vi "Pick&Place_module_cwshih_v0.vi"() -> ()   [LabVIEW 2016]
uses:
  Classes/Controllers/I-O/Copy of NI-DAQ Folder/NI-DAQ.lvclass
  Classes/Controllers/Dispenser/Copy of Ultimus V2 Folder/Ultimus V2.lvclass
  <vilib>/Analysis/coordinate.llb/2D Cartesian Coordinate Rotation (Scalar).vi
  <vilib>/Utility/file.llb/Read Delimited Spreadsheet (DBL).vi
  <vilib>/Utility/file.llb/Write Delimited Spreadsheet (DBL).vi
  Classes/Controllers/Motion/Copy of Motion Folder/Motion.lvclass
  Classes/Controllers/Camera/Copy of Controller Folder/Controller.lvclass
  <vilib>/Analysis/NI_AALPro.lvlib
panel:
  in  "pick up tool measure-start position":dbl[][](array[numeric])=[[147.788, 950.417, 41.7586, -0.0547592], [928.094, 802.097, 34.9367, -0.0626817]]
  out "Array 2":dbl[][](array[numeric])
  out "Measured PickupTool position":dbl[][](array[numeric])
  in  "sampe vacuum":i32[](array[numeric])=[13, 19]
  in  "VacChannel for sample":i32=1
  in  "Values":bool[](array[boolean])=[FALSE, FALSE]
  in  "TrayVaccum":bool
  in  "check height? 2":bool
  in  "check height?":bool
  out "Needle parking position":dbl[](array[numeric])
  out "GlueBox":dbl[][](array[numeric])
  out "appended array":dbl[][](array[numeric])
  in  "chip placement height compensation":dbl=-0.38 format="%#_13g"
  out "Array":dbl[][](array[numeric])
  in  "Sensor A/B":bool
  out "Gantry current position":dbl[](array[numeric])
  in  "READ Position":bool
  in  "Needle Height Compenstation\n(glue gap)":dbl=0.34
  in  "Needle Alignment":bool
  in  "Parking position":dbl[](array[numeric])=[625.0, 625.0, 0.0, 0.01]
  in  "GOTO":bool
  in  "Default Pickup Tool Position":dbl[][](array[numeric])=[[147.788, 950.417, 41.7586, -0.0547592], [928.094, 802.097, 34.9367, -0.0626817]]
  in  "Number of Chips/Sensors \nto be assembled":i32=1
  in  "Default HDI alignment \nmark position":dbl[](array[numeric])=[292.478, 992.407, 78.997, -0.0002369]
  in  "Default HDI size":dbl[](array[numeric])=[24.356, 231.316, -0.0919974, -0.0002369]
  out "# of tasks excuted":i32
  out "Chips on tray position":dbl[][](array[numeric])
  out "measured HDI size":dbl[](array[numeric])
  in  "Chip tray":dbl[](array[numeric])=[388.127, 634.888, 84.693, -0.0231917]
  out "Sample position \non HDI":dbl[][](array[numeric])
  in  "Inititalize":bool
  in  "Pick and place":bool
  in  "Deposit Glue":bool
  in  "Measure Pickup Tools":bool
  in  "Measure Samples on tray":bool
  out "default chip and sensor position w.r.t. 1st mark":dbl[][](array[numeric])
  in  "Assembly Type":bool=TRUE
  in  "Stop":bool
  in  "Measure HDI":bool
  out "Measure HDI top-left":dbl[](array[numeric])
  # "Sensor Tray \nVacuum Channel"
  # "Chips"
  # "Sensor 0.3 -> 200 micron glue thickness\nChips 0.34-> 150 micron glue thickness"
  # "Sensors"
  # "Sensor B short"
  # "Sensors B\n(Short)"
  # "Sensors A\n(Long)"
  # "Sensor A long"
  # "Chips : -0.37-> 60 micron height gap\nSensors (feet stops the lowering)"
  # "ACTIONS"
  # "HDI infomation"
  # "chips use channel 0, 2\nsensors use channel 0, 1"
  # "sensor height 69.8471\nchip height 84.693"
  # "Pick and Place"
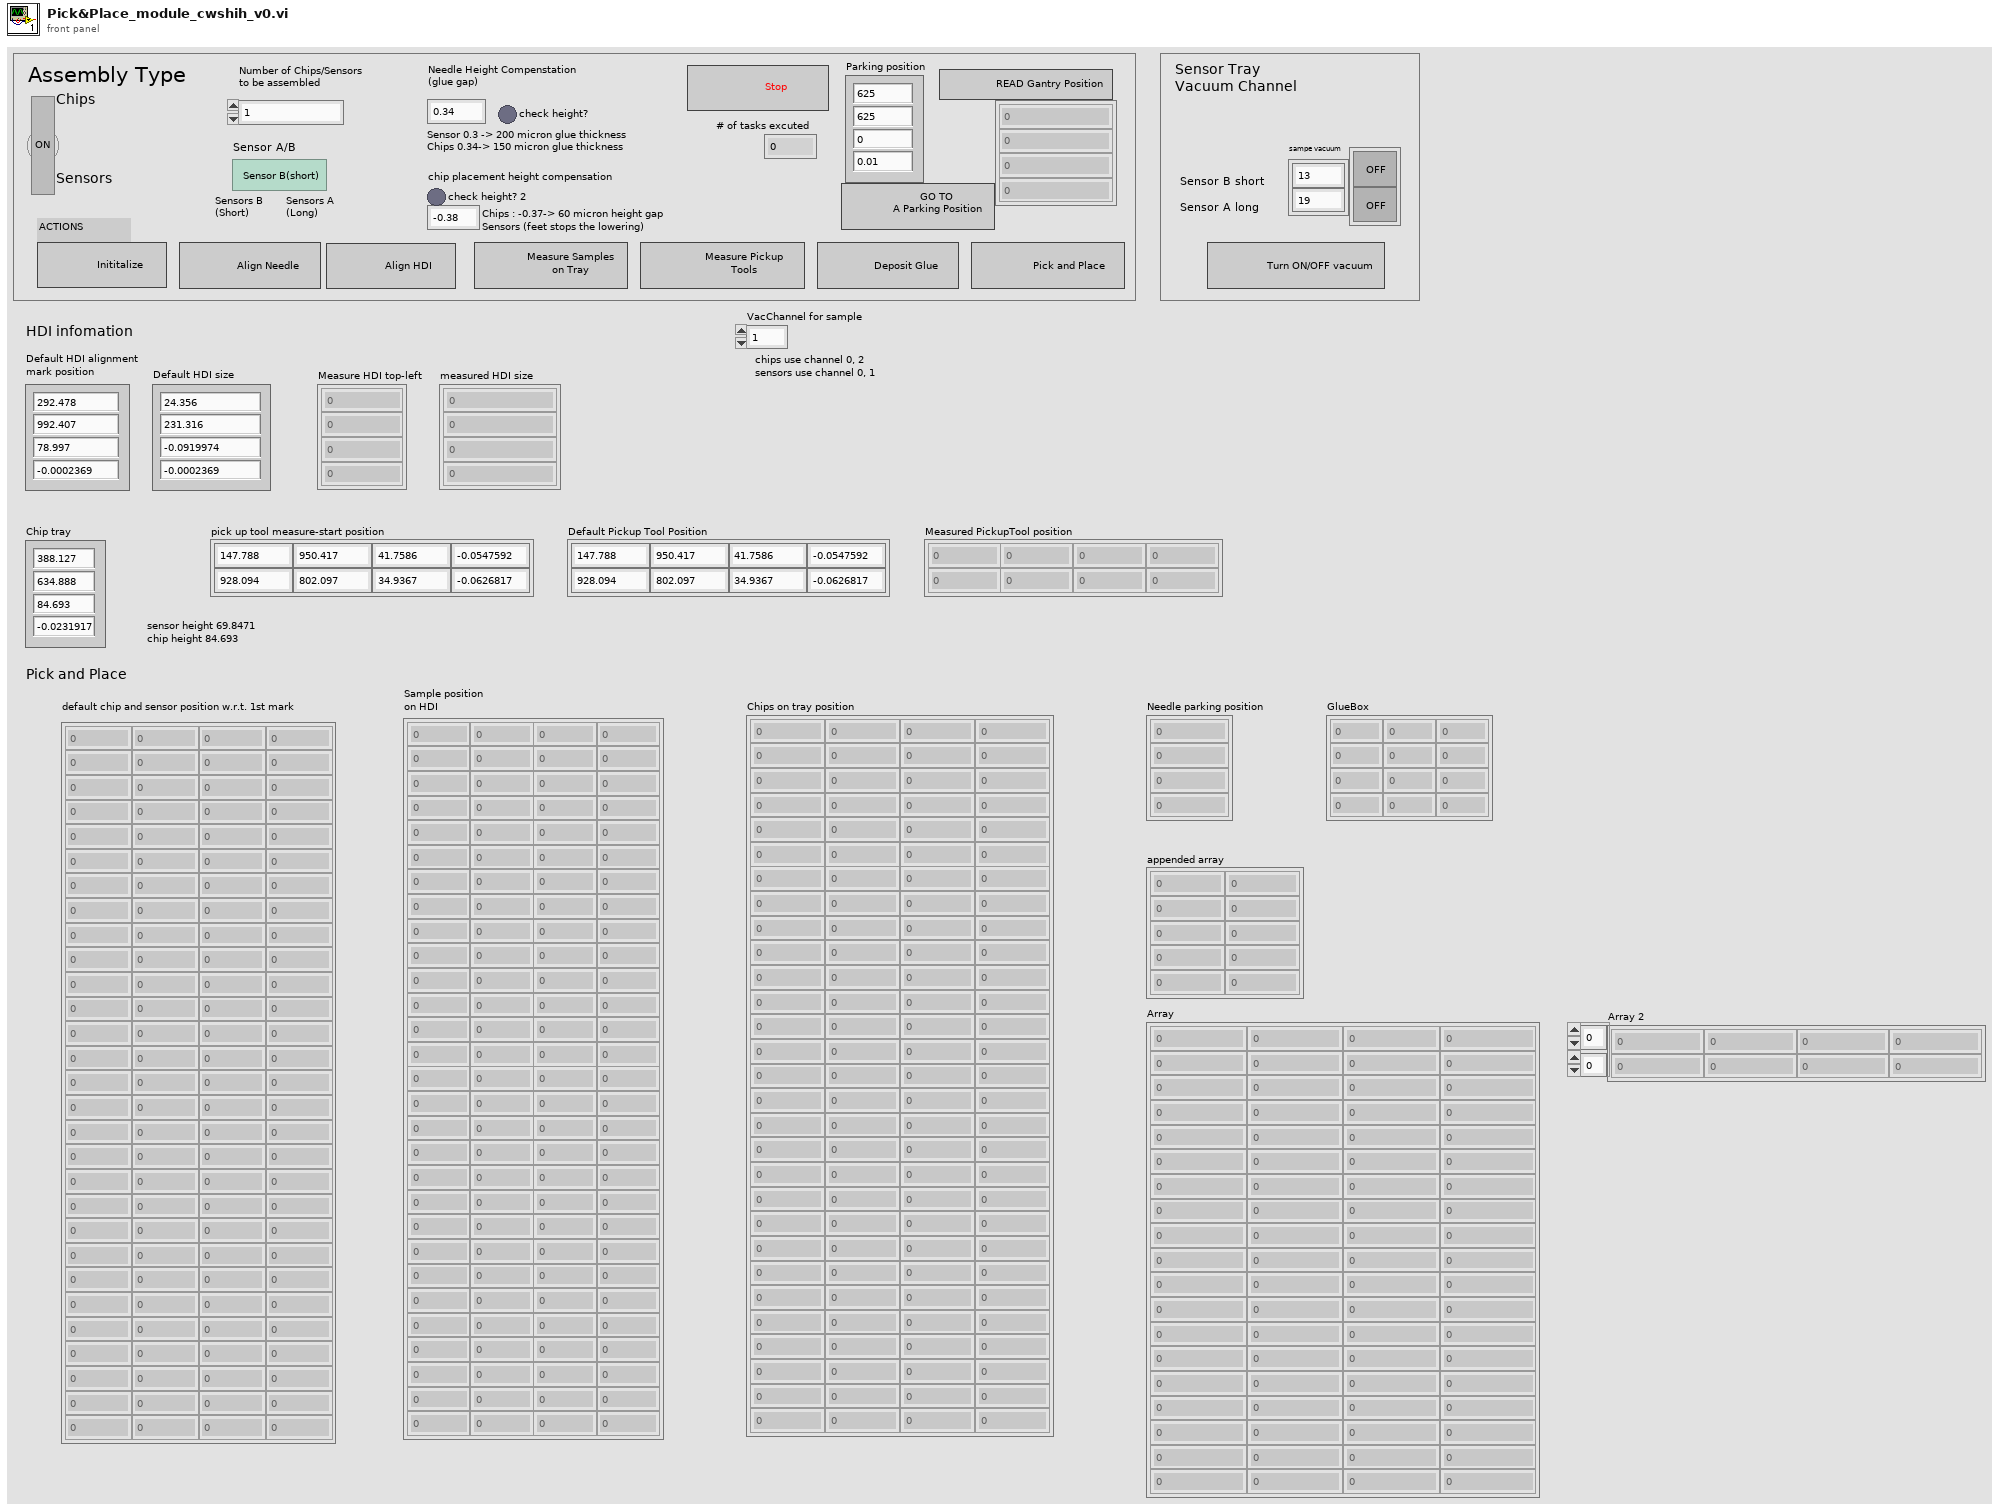
[diagram p1: front panel]
types:
  T1 = typedef "Controller.lvclass/Controllers.ctl" = cluster{"Copy of Motion.lvclass":refnum<class "Motion.lvclass">, "Copy of I-O.lvclass":refnum<class "I-O.lvclass">, "Copy of Dispenser.lvclass":refnum<class "Dispenser.lvclass">}
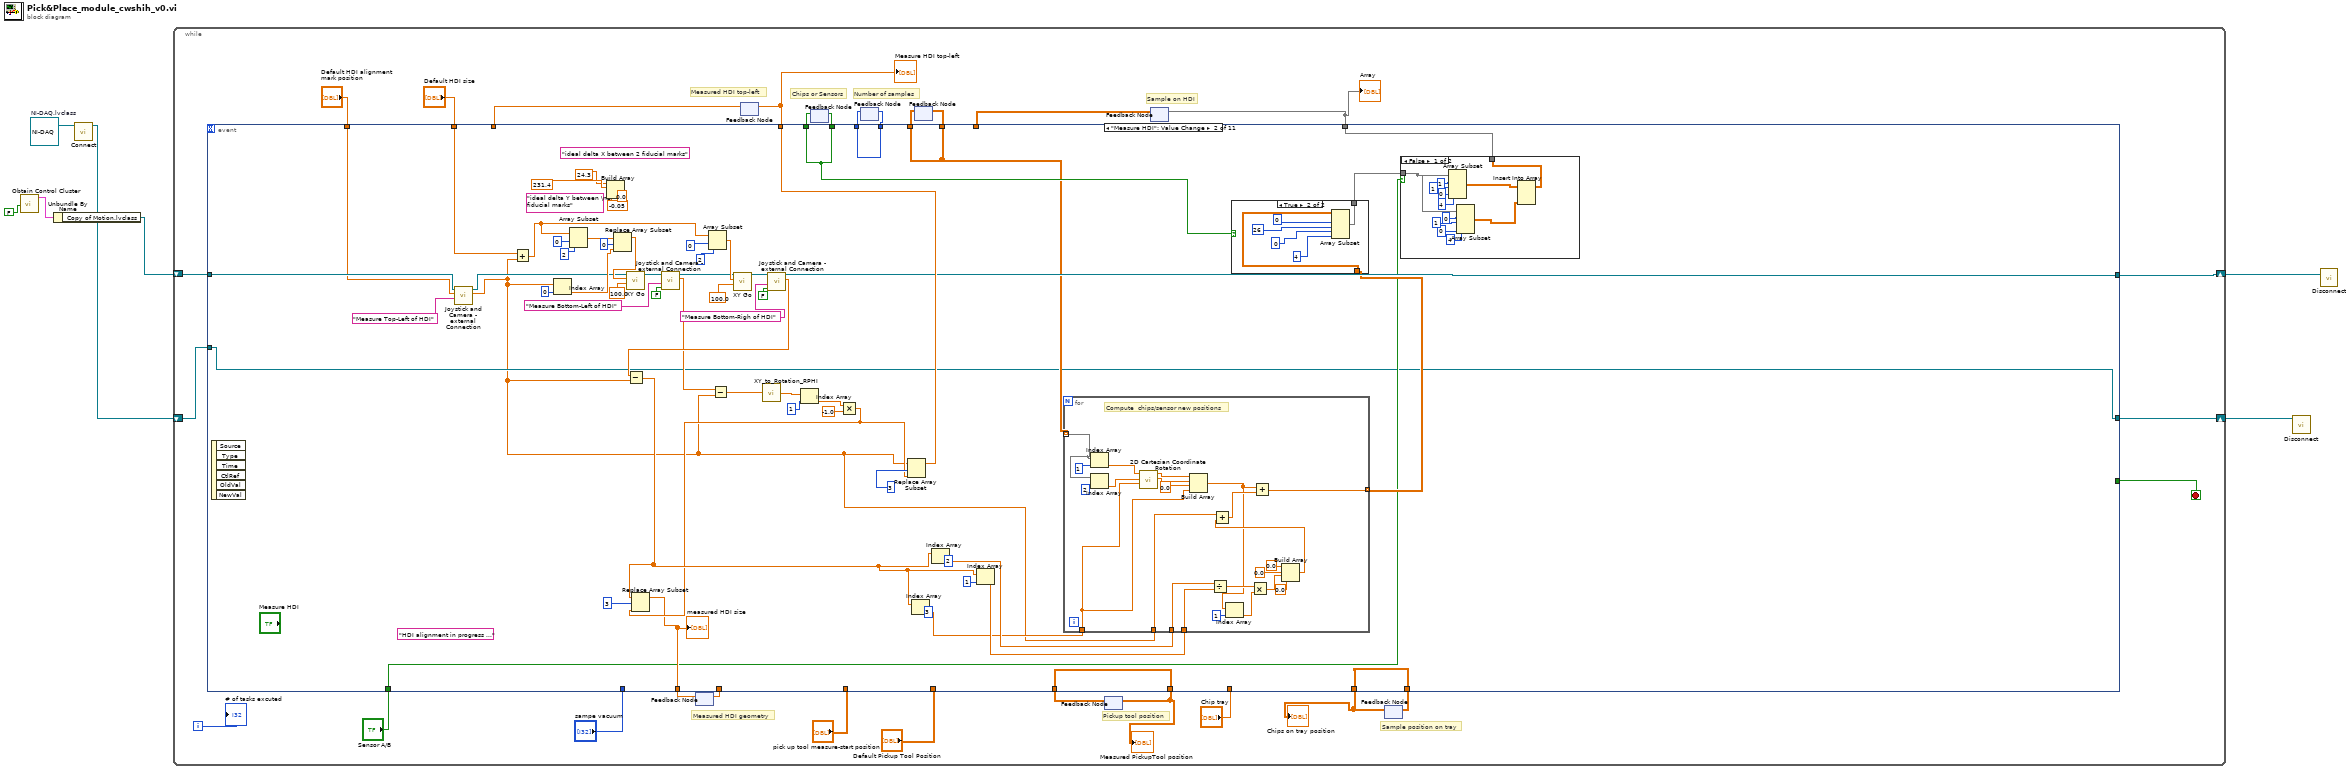
[diagram p0: block diagram]
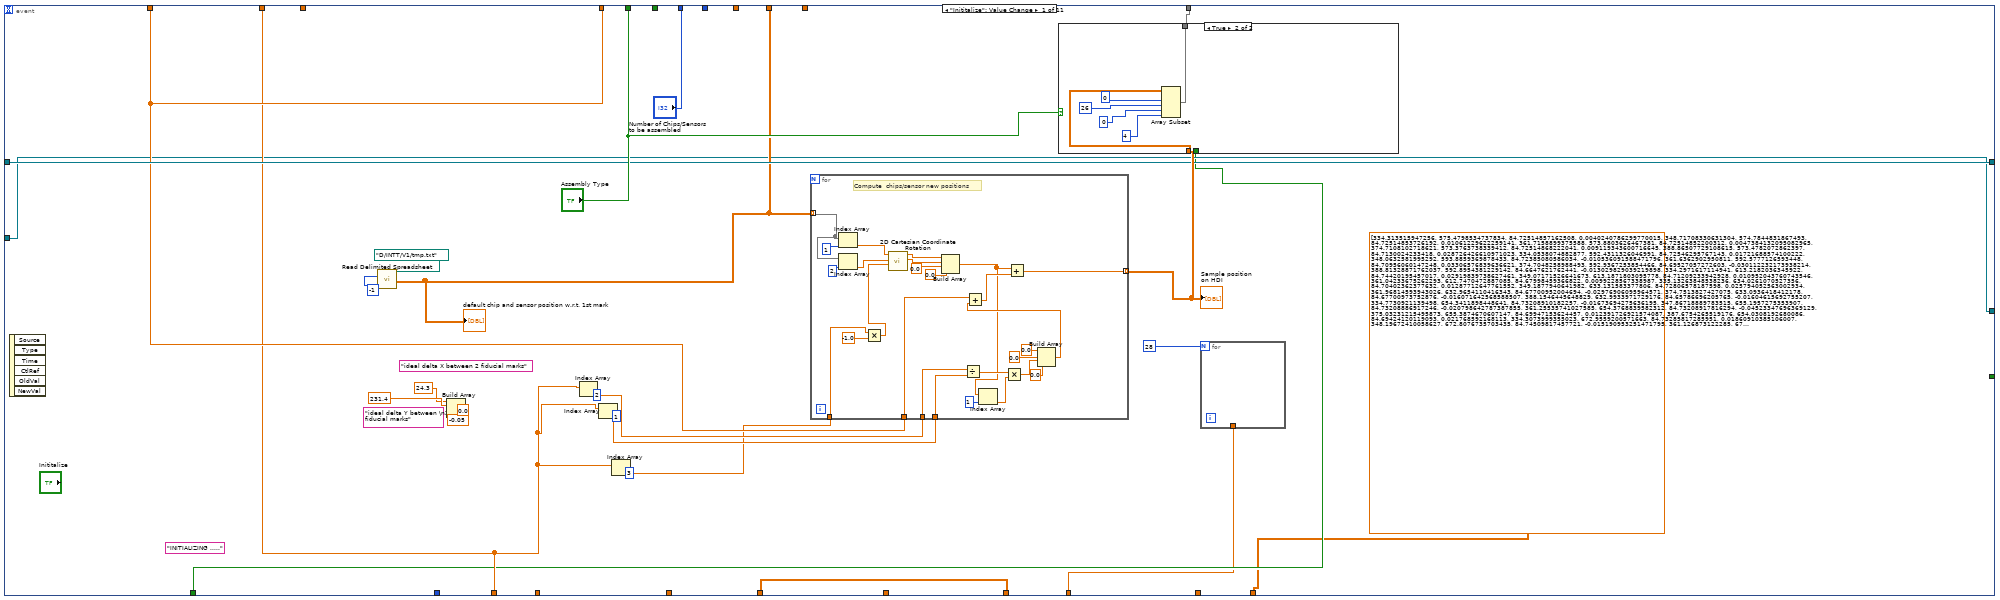
[diagram p2: hidden frame]
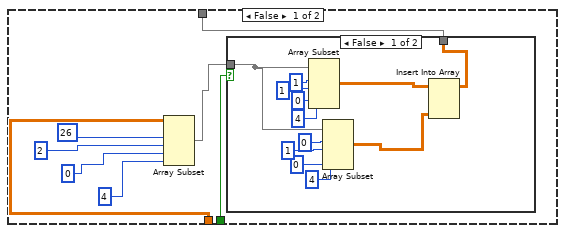
[diagram p3: hidden frame]
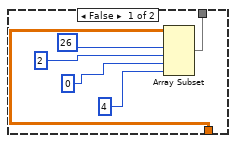
[diagram p6: hidden frame]
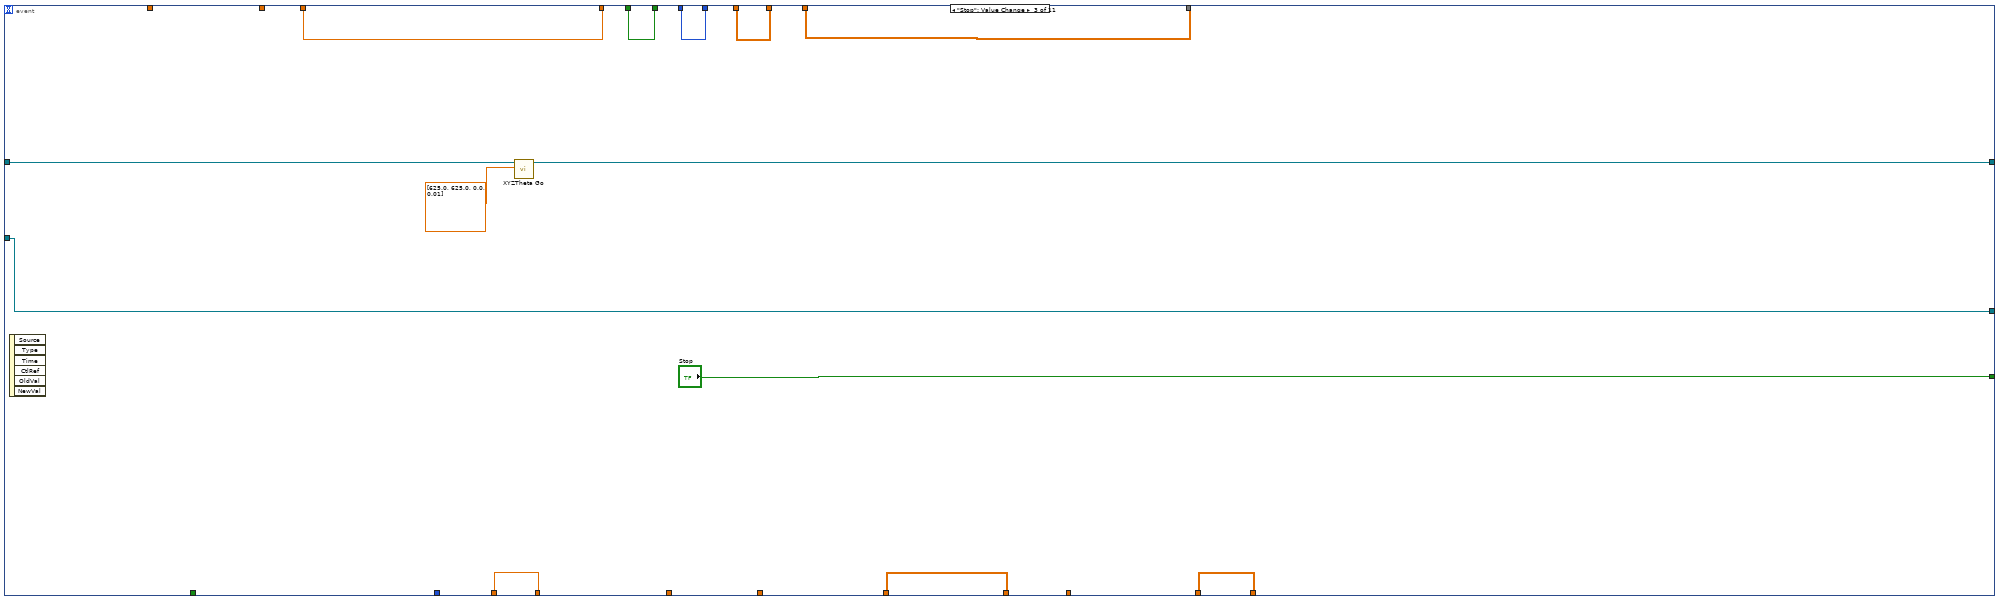
[diagram p7: hidden frame]
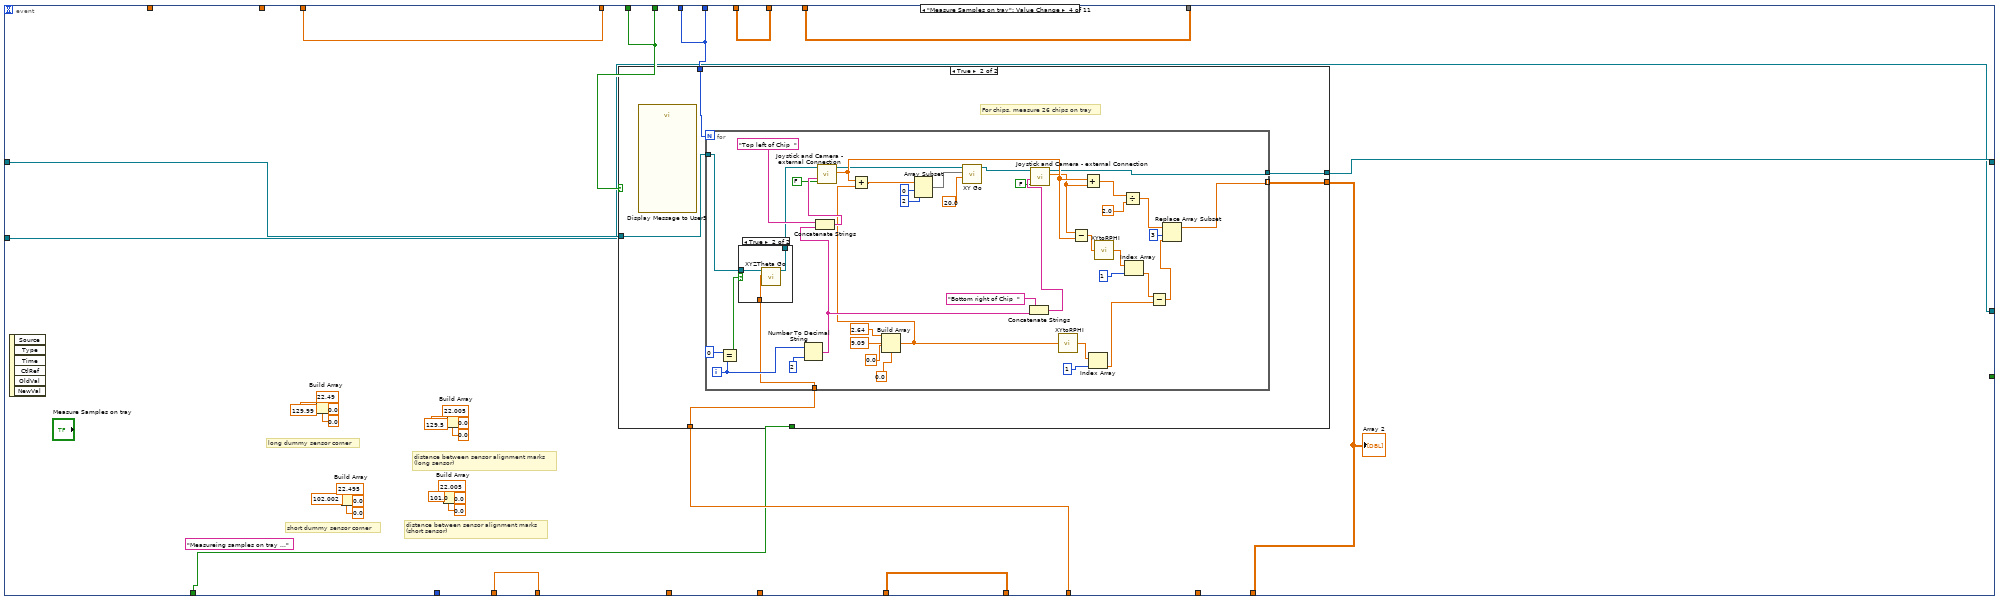
[diagram p8: hidden frame]
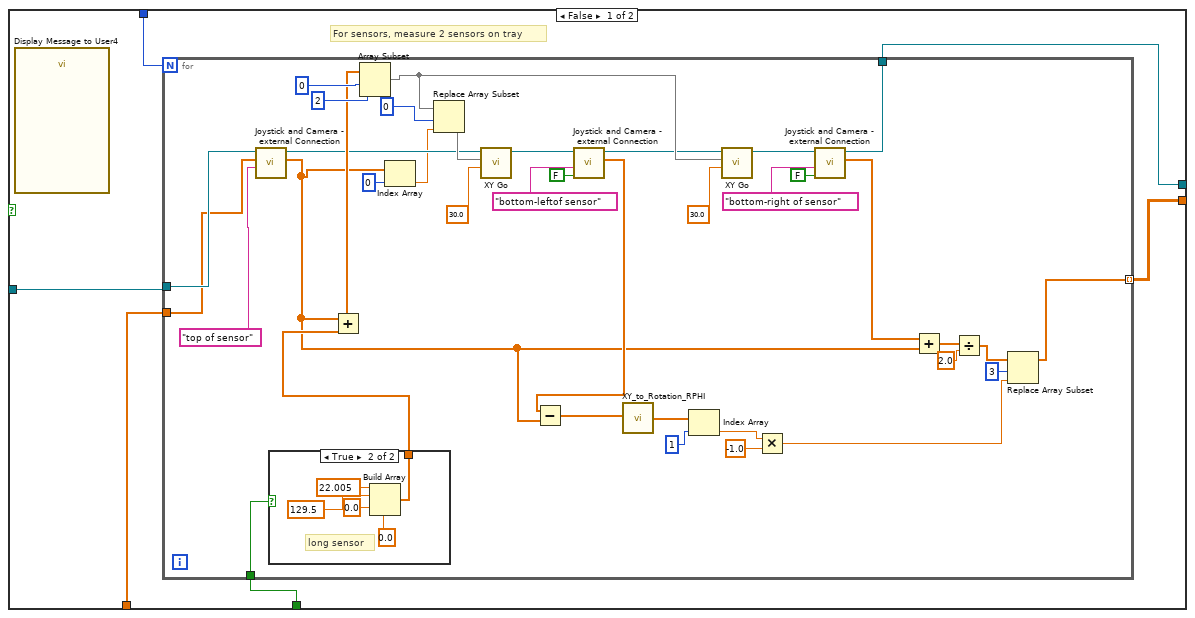
[diagram p9: hidden frame]
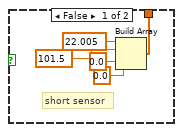
[diagram p10: hidden frame]
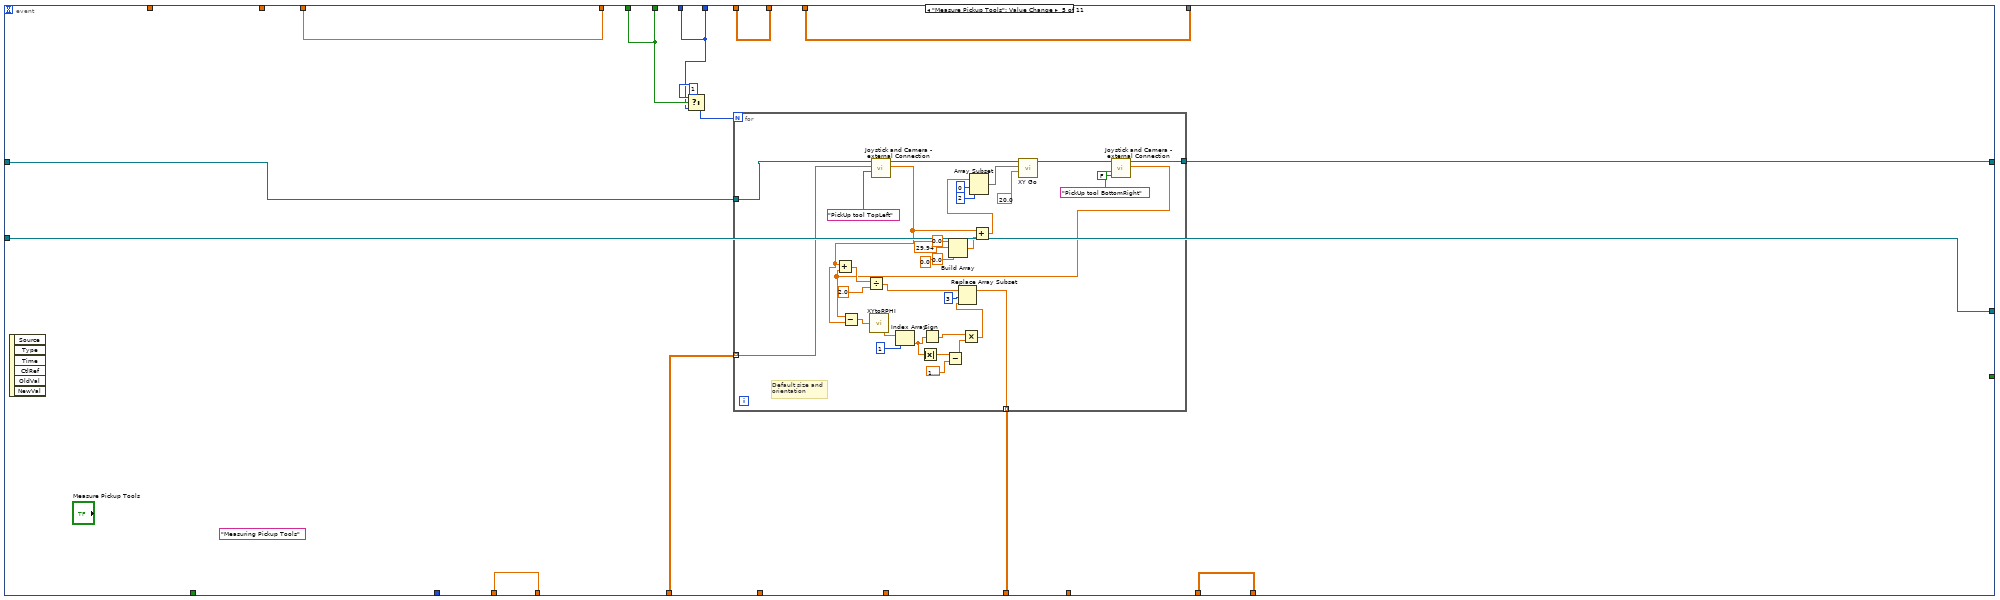
[diagram p12: hidden frame]
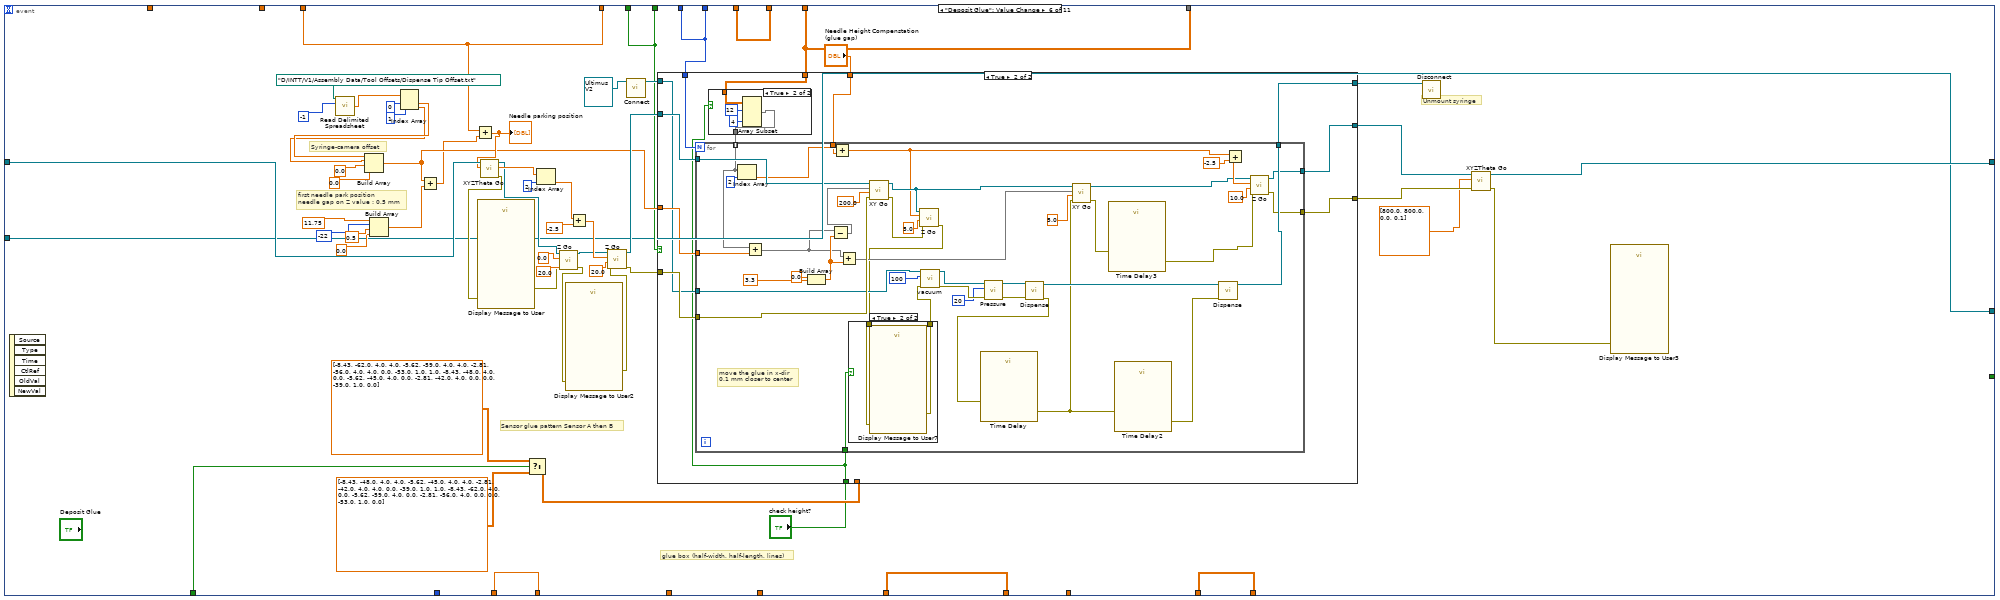
[diagram p13: hidden frame]
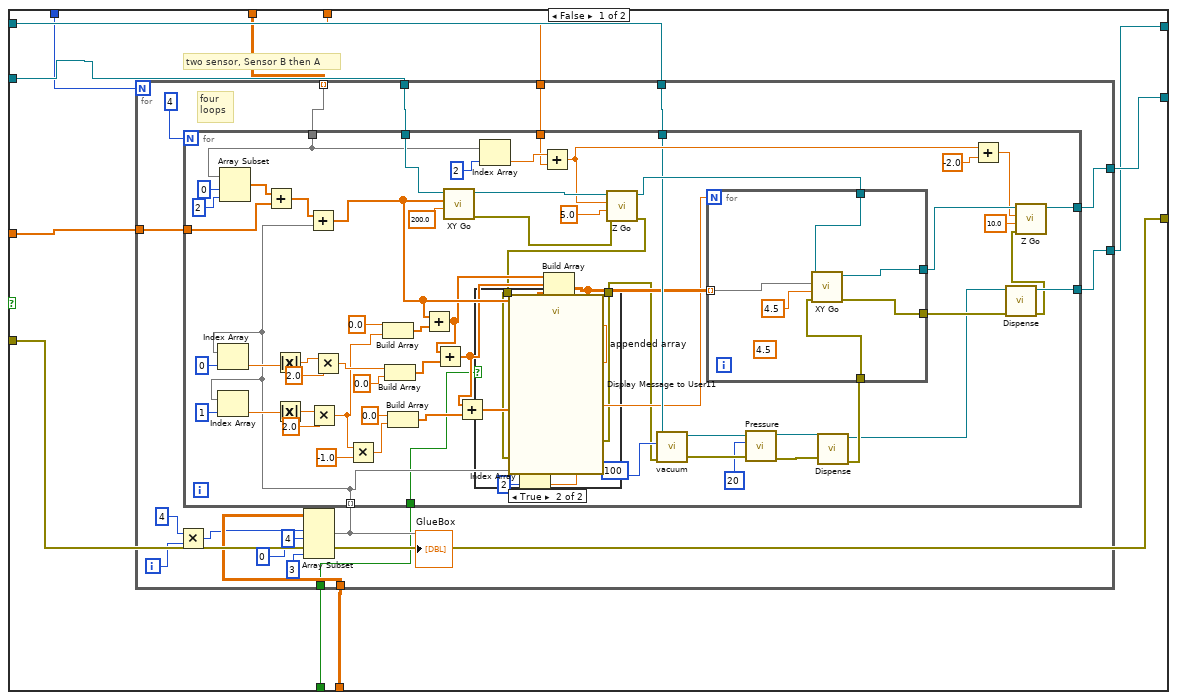
[diagram p14: hidden frame]
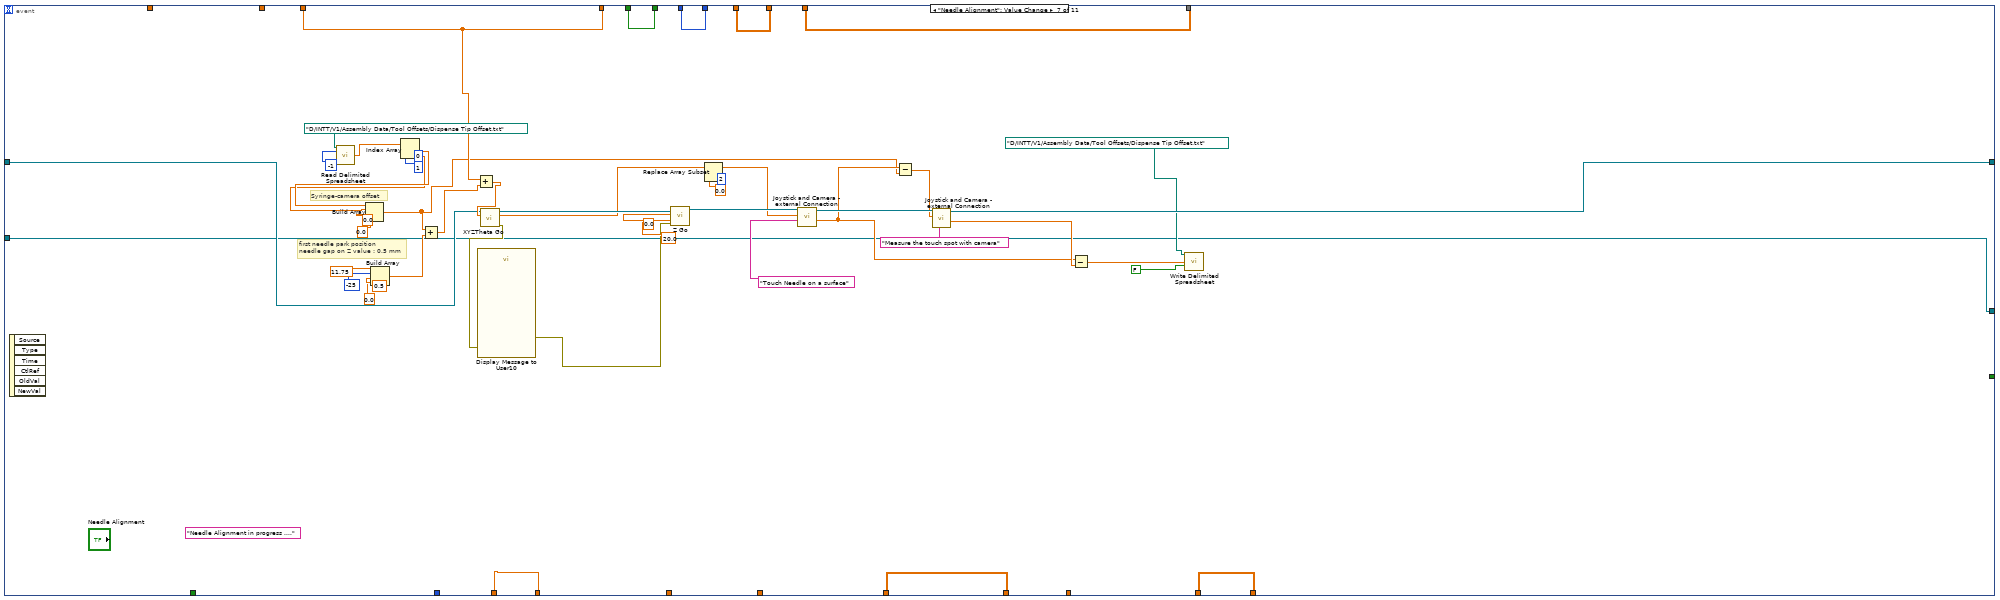
[diagram p18: hidden frame]
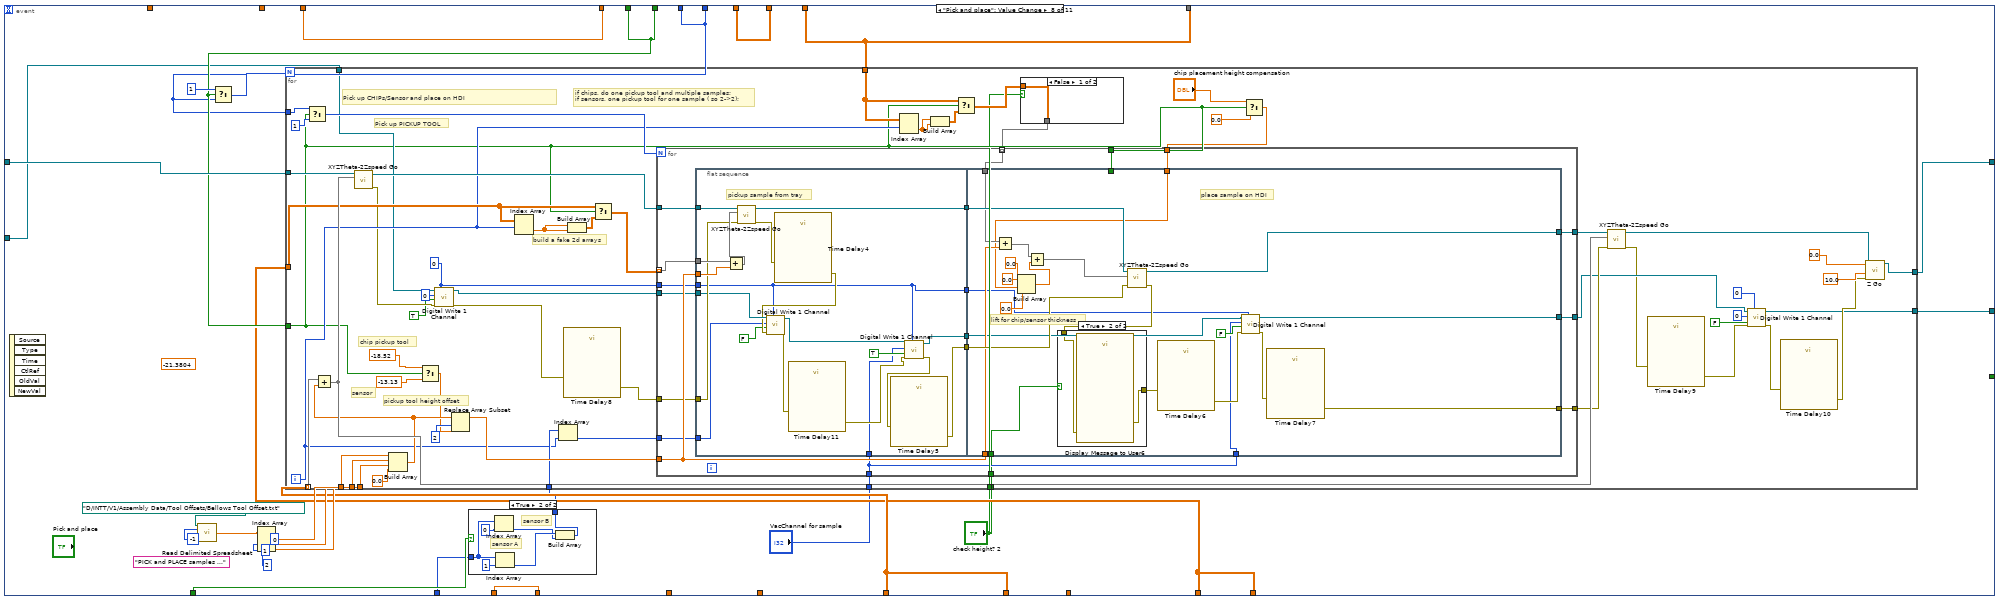
[diagram p19: hidden frame]
diagram:
  w3 = refnum<class "NI-DAQ.lvclass"> refnum  # NI-DAQ.lvclass
  n1 = call "Obtain Control Cluster.vi"("I/O"=FALSE) -> ("Control Out"=w7:T1)  [unwired: 10 in]
  n2 = Unbundle By Name(w7) -> ("Copy of Motion.lvclass"=w5:refnum<class "Motion.lvclass">)
  n3 = call-dynamic "Connect.vi"("NI-DAQ in"=w3) -> ("NI-DAQ out"=w2:refnum<class "NI-DAQ.lvclass">)  [unwired: 9 in, 1 out]
  n4 = while {
    shift-right: [w25] -> w4
    shift-left: w5 -> [w36]
    shift-right: [w12] -> w1
    shift-left: w2 -> [w13]
    i -> [w24]
    stop <- w35 stop-if-true
    # "Pickup tool position"
    # "Chips or Sensors"
    # "Number of samples"
    # "Measured HDI geometry"
    # "Sample position on tray"
    # "Measured HDI top-left"
    # "Sample on HDI"
    n5 = feedback #1() -> (w31:dbl[])  [unwired: 1 in]
    n6 = feedback #2() -> (w33:dbl[])  [unwired: 1 in]
    n7 = feedback #3() -> (w28:bool)  [unwired: 1 in]
    n8 = feedback #4() -> (w23:i32)  [unwired: 1 in]
    n9 = feedback #5() -> (w18:dbl[][])  [unwired: 1 in]
    n10 = feedback #6() -> (w26:dbl[][])  [unwired: 1 in]
    n11 = feedback #7() -> (w30:dbl[][])  [unwired: 1 in]
    n12 = feedback #8() -> (w16:dbl[][])  [unwired: 1 in]
    "Chips on tray position" <- w16
    n13 = event shown="[1] \"Measure HDI\": Value Change" {
      selector: _ -> [_ _ _ _ _ _ _ _ _ _ _]
      dyn-events: _ -> [_ _ _ _ _ _ _ _ _ _ _]
      timeout: _ -> [_ _ _ _ _ _ _ _ _ _ _]
      tunnel: w36 -> [w49 w120 w236 w265 w383 w450 w654 w709 w850 w871 w885]
      tunnel: [_ _ "Stop" _ _ _ _ _ _ _ _] -> w35
      tunnel: [w46 w173 w229 w259 w375 w431 w662 w692 w859 w865 w881] -> w34
      tunnel: w33 -> [_ _ w229 w259 w375 w431 w662 w692 w859 w865 w881]
      tunnel: ["Assembly Type" w166 w233 w263 w379 w434 w661 w698 w858 w866 w882] -> w29
      tunnel: [w44 w125 w228 w258 w374 w427 w657 w691 w854 w864 w880] -> w32
      tunnel: w31 -> [_ _ w228 w258 w374 w427 w657 w691 w854 w864 w880]
      tunnel: [w41 w123 w230 w260 w377 w433 w658 w697 w855 w869 w884] -> w14
      tunnel: w30 -> [_ _ w230 w260 w377 w433 w658 w697 w855 w869 w884]
      tunnel: w28 -> [_ w166 w233 w263 w379 w434 w661 w698 w858 w866 w882]
      tunnel: w23 -> [_ w163 w232 w262 w378 w432 w660 w694 w857 w867 w877]
      tunnel: [dbl[][] [[334.313515947256, 575.4798534737834, 84.72514857162508, 0.0040240786299770015], [348.71708330631304, 574.7844831867493, 84.72514853726192, 0.01061229622259141], [361.7158899375588, 573.8803626467381, 84.72514852200312, 0.0047384132095082965], [374.7108102718621, 573.3763738339412, 84.72514868222041, 0.009119343600716645], [388.86507729108615, 573.4782072862397, 84.7130024233418, 0.028726426610971023], [334.0538074882877, 592.4311326046991, 84.72546295767143, 0.01721688574100222], [348.0632581995292, 593.8859369878433, 84.72385080586034, -0.010536091588471796], [361.6362902950811, 592.5777126593448, 84.70956060147248, 0.03306576839636621], [374.7048258988493, 592.9367253854466, 84.69527057272603, -0.030112232173938214], [388.81328871762037, 592.8954381229142, 84.6647621762441, -0.013029829039219898], [334.2971617114941, 613.2182036345922, 84.74420195457017, 0.02919839738627461], [349.07171526641673, 613.1871803095778, 84.71209233942928, 0.010952043760743546], [361.04233675262293, 612.7470472887085, 84.67998459366822, 0.0099228567338987], [335.13263848538236, 634.0261070527356, 84.70402362377632, 0.01287712647761552], [349.1877940641982, 633.131583377806, 84.72806578187598, 0.025794052563002934], [361.96814593943026, 632.9654110416343, 84.67700952004694, -0.02976906095964571], [374.7513827427075, 633.0936418412178, 84.67700973752876, -0.016071642568588507], [388.1546445648829, 632.9933971729176, 84.65786696205765, -0.01604615692755207], [334.7730921139498, 654.3411898448641, 84.73208910182257, -0.01673694275636195], [347.86718889783515, 655.1957275353907, 84.73208886917246, -0.020798642787387855], [361.25535741027585, 654.3768839582312, 84.73208917816294, -0.04523347696369129], [375.03231215495873, 655.3874670607147, 84.69947153624457, 0.012391726921574087], [387.6754265519176, 654.0308192680086, 84.69424120119093, 0.021768592168113], [334.3073999355023, 672.9559200571663, 84.73285817285951, 0.01860910385106007], [348.19672410058627, 672.8076735703435, 84.74509817457721, -0.015190953251471795], [361.126873122285, 672.7320047678002, 84.74509773207234, -0.005257017136958586]] ("Chips on tray position") w161 w226 w238 w373 w429 w655 w695 w852 w862 w878] -> w27
      tunnel: w16 -> [_ w161 w226 _ w373 w429 w655 w695 w852 w862 w878]
      tunnel: [w39 w162 w227 w257 w382 w428 w656 w696 w853 w863 w879] -> w8
      tunnel: w26 -> [_ w162 w227 w257 _ w428 w656 w696 w853 w863 w879]
      tunnel: [w49 w172 w234 w264 w381 w435 w646 w699 w849 w870 w885] -> w25
      tunnel: ["Number of Chips/Sensors \nto be assembled" w163 w232 w262 w378 w432 w660 w694 w857 w867 w877] -> w22
      tunnel: "Default HDI alignment \nmark position" -> [w46 w116 _ _ _ _ _ _ _ _ _]
      tunnel: "Default HDI size" -> [w44 w171 _ _ _ _ _ _ _ _ _]
      tunnel: [w47 w164 w231 w261 w376 w426 w659 w693 w856 w868 w883] -> w19
      tunnel: w18 -> [_ w164 w231 w261 w376 w426 w659 w693 w856 w868 w883]
      tunnel: "Chip tray" -> [w38 _ _ w256 _ _ _ _ _ _ _]
      tunnel: "Sensor A/B" -> [w40 w122 _ w247 _ w425 _ w690 _ _ _]
      tunnel: w13 -> [w42 w121 w224 w237 w372 w419 w637 w687 w851 w860 w876]
      tunnel: [w42 w121 w224 w237 w372 w419 w637 w688 w851 w860 w875] -> w12
      tunnel: "sampe vacuum" -> [_ _ _ _ _ _ _ w685 _ _ w872]
      tunnel: "Default Pickup Tool Position" -> [w39 _ _ _ _ _ _ _ _ _ _]
      tunnel: "pick up tool measure-start position" -> [_ _ _ _ w371 _ _ _ _ _ _]
      event "Inititalize": Value Change {
        (unwired) "INITIALIZING ....." ("String")
        (unwired) "ideal delta Y between \n2 fiducial marks"
        (unwired) "ideal delta X between 2 fiducial marks"
        n14 = event-data() -> ()  [unwired: 1 in, 6 out]
        n15 = call-poly <vilib>:"Read Delimited Spreadsheet.vi"("file path (dialog if empty)"=path "D:/INTT/V1/tmp.txt", "number of rows (all:-1)"=-1) -> ("all rows"=w47:dbl[][])  [unwired: 8 in, 5 out]
        "default chip and sensor position w.r.t. 1st mark" <- w47
        n16 = Build Array(24.3 ("y"), 231.4 ("y"), 0.0 ("element"), -0.05 ("element")) -> ()  [unwired: 1 out]
        n17 = Index Array(array=w44, index=2) -> (element=w58:dbl)
        n18 = Index Array(array=w44, index=1) -> (element=w57:dbl)
        n19 = Index Array(array=w44, index=3) -> (element=w43:dbl)
        n20 = for {
          tunnel: w47 -> [w108] mode=indexing
          tunnel: w43 -> [w91]
          tunnel: w46 -> [w100]
          tunnel: [w107] -> w51 mode=indexing
          tunnel: w58 -> [w106]
          tunnel: w57 -> [w97]
          # "Compute  chips/sensor new positions"
          n21 = Index Array(array=w108, index=1) -> (element=w112:dbl)
          n22 = Index Array(array=w108, index=2) -> (element=w111:dbl)
          n23 = Multiply(x=w91, y=-1.0) -> (x*y=w90:dbl)
          n24 = call-poly <vilib>:"2D Cartesian Coordinate Rotation.vi"("theta"=w90, "y"=w111, "x"=w112) -> ("y out"=w114:dbl, "x out"=w113:dbl)  [unwired: 6 in, 1 out]
          n25 = Build Array(w113, w114, 0.0 ("element"), 0.0 ("element")) -> (w94:dbl[])
          n26 = Divide(x=w106, y=w97) -> (x/y=w105:dbl)
          n27 = Index Array(array=w94, index=1) -> (element=w95:dbl)
          n28 = Multiply(x=w105, y=w95) -> (x*y=w101:dbl)
          n29 = Build Array(0.0 ("element"), 0.0 ("element"), w101, 0.0 ("element")) -> (w99:dbl[])
          n30 = Add(x=w100, y=w99) -> (x+y=w98:dbl[])
          n31 = Add(x=w94, y=w98) -> (x+y=w107:dbl[])
        }
        "Sample position \non HDI" <- w51
        n32 = case shown="True" "Assembly Type" {
          tunnel: w51 -> [w66 w86]
          tunnel: [w64 w84] -> w41
          tunnel: w40 -> [w63 _]
          frame False {
            n33 = Array Subset(array=w66, index (row)=26 ("index"), length (row)=2 ("length"), index (col)=0, length (col)=4 ("length")) -> (w65:dbl[][])
            n34 = case shown="False" w63 {
              tunnel: w65 -> [w74 w83]
              tunnel: [w71 w83] -> w64
              frame False {
                n35 = Array Subset(array=w74, index (row)=1 ("index"), length (row)=1 ("length"), index (col)=0 ("index"), length (col)=4 ("length")) -> (w73:dbl[][])
                n36 = Array Subset(array=w74, index (row)=0 ("index"), length (row)=1 ("length"), index (col)=0 ("index"), length (col)=4 ("length")) -> (w72:dbl[][])
                n37 = Insert Into Array(array=w73, new element=w72) -> (w71:dbl[][])  [unwired: 2 in]
              }
              frame True {
              }
            }
          }
          frame True {
            n38 = Array Subset(array=w86, index (row)=0 ("index"), length (row)=26 ("length"), index (col)=0, length (col)=4 ("length")) -> (w84:dbl[][])
          }
        }
        n39 = for {
          N: 28 -> [_]
          tunnel: w38 -> [_]
        }
      }
      event "Measure HDI": Value Change {
        (unwired) "ideal delta Y between \n2 fiducial marks"
        (unwired) "ideal delta X between 2 fiducial marks"
        (unwired) "HDI alignment in progress ..." ("String")
        n40 = event-data() -> ()  [unwired: 1 in, 6 out]
        n41 = call "Joystick and Camera - external Connection.vi"("Motion in"=w120, "XYZTheta"=w116, "Measurement Point"="Measure Top-Left of HDI") -> ("Motion out"=w119:refnum<class "Motion.lvclass">, "Sum"=w118:dbl[])  [unwired: 4 in, 2 out]
        n42 = Add(x=w171, y=w118) -> (x+y=w143:dbl[])
        n43 = Index Array(array=w118, index=0) -> (element=w132:dbl)
        n44 = Array Subset(array=w143, index=0, length=2) -> (w142:dbl[])
        n45 = Build Array(24.3 ("y"), 231.4 ("y"), 0.0 ("element"), -0.05 ("element")) -> ()  [unwired: 1 out]
        n46 = Replace Array Subset(array=w142, new element=w132, index=0) -> (w140:dbl[])
        n47 = call-dynamic "XY Go.vi"("Speed"=100.0, "XY"=w140, "Motion in"=w119) -> ("Motion out"=w147:refnum<class "Motion.lvclass">)  [unwired: 7 in, 1 out]
        n48 = call "Joystick and Camera - external Connection.vi"("Motion in"=w147, "Measurement Point"="Measure Bottom-Left of HDI", "Inital GO"=FALSE) -> ("Motion out"=w139:refnum<class "Motion.lvclass">, "Sum"=w131:dbl[])  [unwired: 4 in, 2 out]
        n49 = Array Subset(array=w143, index=0, length=2) -> (w153:dbl[])
        n50 = Subtract(x=w131, y=w118) -> (x-y=w138:dbl[])
        n51 = call-dynamic "XY Go.vi"("Speed"=100.0, "XY"=w153, "Motion in"=w139) -> ("Motion out"=w157:refnum<class "Motion.lvclass">)  [unwired: 7 in, 1 out]
        n52 = call "XY_to_Rotation_RPHI.vi"("X-Y"=w138) -> ("r-phi"=w135:dbl[])
        n53 = call "Joystick and Camera - external Connection.vi"("Motion in"=w157, "Measurement Point"="Measure Bottom-Righ of HDI", "Inital GO"=FALSE) -> ("Motion out"=w172:refnum<class "Motion.lvclass">, "Sum"=w175:dbl[])  [unwired: 4 in, 2 out]
        n54 = Subtract(x=w175, y=w118) -> (x-y=w128:dbl[])
        n55 = Index Array(array=w135, index=1) -> (element=w129:dbl)
        n56 = Multiply(x=w129, y=-1.0) -> (x*y=w126:dbl)
        n57 = Replace Array Subset(array=w128, new element=w126, index=3) -> (w125:dbl[])
        "measured HDI size" <- w125
        n58 = Replace Array Subset(array=w118, new element=w126, index=3) -> (w173:dbl[])
        n59 = Index Array(array=w128, index=3) -> (element=w159:dbl)
        n60 = Index Array(array=w128, index=2) -> (element=w168:dbl)
        n61 = Index Array(array=w128, index=1) -> (element=w167:dbl)
        n62 = for {
          tunnel: w164 -> [w216] mode=indexing
          tunnel: w159 -> [w201]
          tunnel: w118 -> [w208]
          tunnel: [w215] -> w165 mode=indexing
          tunnel: w168 -> [w214]
          tunnel: w167 -> [w205]
          # "Compute  chips/sensor new positions"
          n63 = Index Array(array=w216, index=1) -> (element=w220:dbl)
          n64 = Index Array(array=w216, index=2) -> (element=w219:dbl)
          n65 = call-poly <vilib>:"2D Cartesian Coordinate Rotation.vi"("theta"=w201, "y"=w219, "x"=w220) -> ("y out"=w222:dbl, "x out"=w221:dbl)  [unwired: 6 in, 1 out]
          n66 = Build Array(w221, w222, 0.0 ("element"), w201) -> (w202:dbl[])
          n67 = Divide(x=w214, y=w205) -> (x/y=w213:dbl)
          n68 = Index Array(array=w202, index=1) -> (element=w203:dbl)
          n69 = Multiply(x=w213, y=w203) -> (x*y=w209:dbl)
          n70 = Build Array(0.0 ("element"), 0.0 ("element"), w209, 0.0 ("element")) -> (w207:dbl[])
          n71 = Add(x=w208, y=w207) -> (x+y=w206:dbl[])
          n72 = Add(x=w202, y=w206) -> (x+y=w215:dbl[])
        }
        n73 = case shown="True" w166 {
          tunnel: w165 -> [w190 w197]
          tunnel: [w189 w195] -> w124
          frame False {
            n74 = Array Subset(array=w190, index (row)=26 ("index"), length (row)=2 ("length"), index (col)=0, length (col)=4 ("length")) -> (w189:dbl[][])
          }
          frame True {
            n75 = Array Subset(array=w197, index (row)=0 ("index"), length (row)=26 ("length"), index (col)=0, length (col)=4 ("length")) -> (w195:dbl[][])
          }
        }
        n76 = case shown="False" w122 {
          tunnel: w124 -> [w179 w188]
          tunnel: [w176 w188] -> w123
          frame False {
            n77 = Array Subset(array=w179, index (row)=1 ("index"), length (row)=1 ("length"), index (col)=0 ("index"), length (col)=4 ("length")) -> (w178:dbl[][])
            n78 = Array Subset(array=w179, index (row)=0 ("index"), length (row)=1 ("length"), index (col)=0 ("index"), length (col)=4 ("length")) -> (w177:dbl[][])
            n79 = Insert Into Array(array=w178, new element=w177) -> (w176:dbl[][])  [unwired: 2 in]
          }
          frame True {
          }
        }
      }
      event "Stop": Value Change {
        n80 = event-data() -> ()  [unwired: 1 in, 6 out]
        n81 = call "XYZTheta Go.vi"("XYZTheta In"=dbl[] [625.0, 625.0, 0.0, 0.01], "Motion in"=w236) -> ("Motion out"=w234:refnum<class "Motion.lvclass">)  [unwired: 7 in, 2 out]
      }
      event "Measure Samples on tray": Value Change {
        (unwired) "Measureing samples on tray ..." ("String")
        # "long dummy sensor corner"
        # "short dummy sensor corner"
        # "distance between sensor alignment marks\n(short sensor)"
        # "distance between sensor alignment marks\n(long sensor)"
        n82 = event-data() -> ()  [unwired: 1 in, 6 out]
        n83 = Build Array(22.49 ("element"), 129.99 ("element"), 0.0 ("element"), 0.0 ("element")) -> ()  [unwired: 1 out]
        n84 = Build Array(22.495 ("element"), 102.002 ("element"), 0.0 ("element"), 0.0 ("element")) -> ()  [unwired: 1 out]
        n85 = Build Array(22.005 ("element"), 101.0 ("element"), 0.0 ("element"), 0.0 ("element")) -> ()  [unwired: 1 out]
        n86 = Build Array(22.005 ("element"), 129.5 ("element"), 0.0 ("element"), 0.0 ("element")) -> ()  [unwired: 1 out]
        n87 = case shown="True" w263 {
          tunnel: [w267 w324] -> w238
          tunnel: w265 -> [w271 w323]
          tunnel: [w266 w322] -> w264
          tunnel: w262 -> [w270 w321]
          tunnel: w256 -> [w269 w320]
          tunnel: w247 -> [w268 _]
          frame False {
            # "For sensors, measure 2 sensors on tray"
            n88 = call "Display Message to User4"() -> ()  [unwired: 10 in, 2 out]
            n89 = for {
              N: w270 -> [_]
              tunnel: w271 -> [w309]
              tunnel: [w306] -> w266
              tunnel: [w299] -> w267 mode=indexing
              tunnel: w269 -> [w298]
              tunnel: w268 -> [w297]
              n90 = call "Joystick and Camera - external Connection.vi"("Motion in"=w309, "XYZTheta"=w298, "Measurement Point"="top of sensor") -> ("Motion out"=w276:refnum<class "Motion.lvclass">, "Sum"=w273:dbl[])  [unwired: 4 in, 2 out]
              n91 = case shown="True" w297 {
                tunnel: [w310 w316] -> w300
                frame False {
                  # "short sensor"
                  n92 = Build Array(22.005 ("element"), 101.5 ("element"), 0.0 ("element"), 0.0 ("element")) -> (w310:dbl[])
                }
                frame True {
                  # "long sensor"
                  n93 = Build Array(22.005 ("element"), 129.5 ("element"), 0.0 ("element"), 0.0 ("element")) -> (w316:dbl[])
                }
              }
              n94 = Add(x=w273, y=w300) -> (x+y=w286:dbl[])
              n95 = Array Subset(array=w286, index=0, length=2) -> (w287:dbl[])
              n96 = Index Array(array=w273, index=0) -> (element=w272:dbl)
              n97 = Replace Array Subset(array=w287, new element=w272, index=0) -> (w284:dbl[])
              n98 = call-dynamic "XY Go.vi"("Speed"=30.0, "XY"=w284, "Motion in"=w276) -> ("Motion out"=w289:refnum<class "Motion.lvclass">)  [unwired: 7 in, 1 out]
              n99 = call "Joystick and Camera - external Connection.vi"("Motion in"=w289, "Measurement Point"="bottom-leftof sensor", "Inital GO"=FALSE) -> ("Motion out"=w275:refnum<class "Motion.lvclass">, "Sum"=w278:dbl[])  [unwired: 4 in, 2 out]
              n100 = Subtract(x=w278, y=w273) -> (x-y=w283:dbl[])
              n101 = call "XY_to_Rotation_RPHI.vi"("X-Y"=w283) -> ("r-phi"=w282:dbl[])
              n102 = Index Array(array=w282, index=1) -> (element=w279:dbl)
              n103 = call-dynamic "XY Go.vi"("Speed"=30.0, "XY"=w287, "Motion in"=w275) -> ("Motion out"=w295:refnum<class "Motion.lvclass">)  [unwired: 7 in, 1 out]
              n104 = Multiply(x=w279, y=-1.0) -> (x*y=w277:dbl)
              n105 = call "Joystick and Camera - external Connection.vi"("Motion in"=w295, "Measurement Point"="bottom-right of sensor", "Inital GO"=FALSE) -> ("Motion out"=w306:refnum<class "Motion.lvclass">, "Sum"=w303:dbl[])  [unwired: 4 in, 2 out]
              n106 = Add(x=w303, y=w273) -> (x+y=w304:dbl[])
              n107 = Divide(x=w304, y=2.0) -> (x/y=w302:dbl[])
              n108 = Replace Array Subset(array=w302, new element=w277, index=3) -> (w299:dbl[])
            }
          }
          frame True {
            # "For chips, measure 26 chips on tray"
            n109 = call "Display Message to User5"() -> ()  [unwired: 10 in, 2 out]
            n110 = for {
              N: w321 -> [_]
              tunnel: [w353] -> w324 mode=indexing
              tunnel: w323 -> [w337]
              tunnel: [w333] -> w322
              tunnel: w320 -> [w338]
              i -> [w341]
              n111 = Equal?(x=0, y=w341) -> (x = y?=w339:bool)
              n112 = case shown="True" w339 {
                tunnel: w338 -> [_ w370]
                tunnel: w337 -> [w367 w369]
                tunnel: [w367 w368] -> w336
                frame False {
                }
                frame True {
                  n113 = call "XYZTheta Go.vi"("XYZTheta In"=w370, "Motion in"=w369) -> ("Motion out"=w368:refnum<class "Motion.lvclass">)  [unwired: 7 in, 2 out]
                }
              }
              n114 = Number To Decimal String(number=w341, width (-)=i16 2) -> (decimal integer string=w357:string)
              n115 = Concatenate Strings("Top left of Chip  " ("string"), w357) -> (w351:string)
              n116 = call "Joystick and Camera - external Connection.vi"("Motion in"=w336, "Measurement Point"=w351, "Inital GO"=FALSE) -> ("Motion out"=w326:refnum<class "Motion.lvclass">, "Sum"=w356:dbl[])  [unwired: 4 in, 2 out]
              n117 = Build Array(2.64 ("element"), 9.09 ("element"), 0.0 ("element"), 0.0 ("element")) -> (w346:dbl[])
              n118 = Add(x=w356, y=w346) -> (x+y=w327:dbl[])
              n119 = Array Subset(array=w327, index=0, length=2) -> (w328:dbl[])
              n120 = call-dynamic "XY Go.vi"("Speed"=20.0, "XY"=w328, "Motion in"=w326) -> ("Motion out"=w325:refnum<class "Motion.lvclass">)  [unwired: 7 in, 1 out]
              n121 = Concatenate Strings("Bottom right of Chip  " ("string"), w357) -> (w335:string)
              n122 = call "Joystick and Camera - external Connection.vi"("Motion in"=w325, "Measurement Point"=w335, "Inital GO"=FALSE) -> ("Motion out"=w333:refnum<class "Motion.lvclass">, "Sum"=w332:dbl[])  [unwired: 4 in, 2 out]
              n123 = call "XYtoRPHI.vi"("X-Y"=w346) -> ("r-phi"=w348:dbl[])
              n124 = Subtract(x=w332, y=w356) -> (x-y=w349:dbl[])
              n125 = Add(x=w356, y=w332) -> (x+y=w363:dbl[])
              n126 = Index Array(array=w348, index=1) -> (element=w343:dbl)
              n127 = call "XYtoRPHI.vi"("X-Y"=w349) -> ("r-phi"=w361:dbl[])
              n128 = Divide(x=w363, y=2.0) -> (x/y=w355:dbl[])
              n129 = Index Array(array=w361, index=1) -> (element=w344:dbl)
              n130 = Subtract(x=w344, y=w343) -> (x-y=w345:dbl)
              n131 = Replace Array Subset(array=w355, new element=w345, index=3) -> (w353:dbl[])
            }
          }
        }
        "Array 2" <- w238
      }
      event "Measure Pickup Tools": Value Change {
        (unwired) "Measuring Pickup Tools" ("String")
        n132 = event-data() -> ()  [unwired: 1 in, 6 out]
        n133 = Select(t=i8 1, s=w379, f=w378) -> (s? t:f=w380:i32)
        n134 = for {
          N: w380 -> [_]
          tunnel: [w408] -> w382 mode=indexing
          tunnel: w383 -> [w412]
          tunnel: [w394] -> w381
          tunnel: w371 -> [w385] mode=indexing
          # "Default size and\norientation"
          n135 = call "Joystick and Camera - external Connection.vi"("Motion in"=w412, "XYZTheta"=w385, "Measurement Point"="PickUp tool TopLeft") -> ("Motion out"=w389:refnum<class "Motion.lvclass">, "Sum"=w411:dbl[])  [unwired: 4 in, 2 out]
          n136 = Build Array(0.0 ("element"), 29.94 ("element"), 0.0 ("element"), 0.0 ("element")) -> (w399:dbl[])
          n137 = Add(x=w411, y=w399) -> (x+y=w386:dbl[])
          n138 = Array Subset(array=w386, index=0, length=2) -> (w387:dbl[])
          n139 = call-dynamic "XY Go.vi"("Speed"=20.0, "XY"=w387, "Motion in"=w389) -> ("Motion out"=w388:refnum<class "Motion.lvclass">)  [unwired: 7 in, 1 out]
          n140 = call "Joystick and Camera - external Connection.vi"("Motion in"=w388, "Measurement Point"="PickUp tool BottomRight", "Inital GO"=FALSE) -> ("Motion out"=w394:refnum<class "Motion.lvclass">, "Sum"=w410:dbl[])  [unwired: 4 in, 2 out]
          n141 = Add(x=w411, y=w410) -> (x+y=w417:dbl[])
          n142 = Subtract(x=w410, y=w411) -> (x-y=w409:dbl[])
          n143 = Divide(x=w417, y=2.0) -> (x/y=w414:dbl[])
          n144 = call "XYtoRPHI.vi"("X-Y"=w409) -> ("r-phi"=w415:dbl[])
          n145 = Index Array(array=w415, index=1) -> (element=w403:dbl)
          n146 = Absolute Value(x=w403) -> (abs(x)=w406:dbl)
          n147 = Sign(1:w403) -> (0:w404:dbl)
          n148 = Subtract(x=w406, y=1.5707963267948966) -> (x-y=w405:dbl)
          n149 = Multiply(x=w404, y=w405) -> (x*y=w402:dbl)
          n150 = Replace Array Subset(array=w414, new element=w402, index=3) -> (w408:dbl[])
        }
      }
      event "Deposit Glue": Value Change {
        # "glue box (half-width, half-length, lines)"
        # "Sensor glue pattern Sensor A then B"
        # "Unmount syringe"
        # "first needle park position\nneedle gap on Z value : 0.5 mm"
        # "Syringe-camera offset"
        n151 = event-data() -> ()  [unwired: 1 in, 6 out]
        n152 = call-poly <vilib>:"Read Delimited Spreadsheet.vi"("file path (dialog if empty)"=path "D:/INTT/V1/Assembly Data/Tool Offsets/Dispense Tip Offset.txt", "number of rows (all:-1)"=-1) -> ("first row"=w470:dbl[])  [unwired: 8 in, 5 out]
        n153 = Build Array(11.75, -22, 0.5 ("element"), 0.0 ("element")) -> (w463:dbl[])
        n154 = Index Array(array=w470, index #1=0 ("index"), index #2=1 ("index")) -> (element #1=w465:dbl, element #2=w462:dbl)
        n155 = Build Array(w465, w462, 0.0 ("element"), 0.0 ("element")) -> (w443:dbl[])
        n156 = Add(x=w443, y=w463) -> (x+y=w430:dbl[])
        n157 = Add(x=w431, y=w430) -> (x+y=w449:dbl[])
        "Needle parking position" <- w449
        n158 = call "XYZTheta Go.vi"("XYZTheta In"=w449, "Motion in"=w450) -> ("error out"=w461:errorcluster, "XYZTheta Out"=w459:dbl[], "Motion out"=w448:refnum<class "Motion.lvclass">)  [unwired: 7 in]
        n159 = call "Display Message to User"("error in (no error)"=w461) -> ("error out"=w451:errorcluster)  [unwired: 9 in, 1 out]
        n160 = Select(t=dbl[][] [[-8.43, -62.0, 4.0, 4.0], [-5.62, -59.0, 4.0, 4.0], [-2.81, -56.0, 4.0, 4.0], [0.0, -53.0, 1.0, 1.0], [-8.43, -48.0, 4.0, 0.0], [-5.62, -45.0, 4.0, 0.0], [-2.81, -42.0, 4.0, 0.0], [0.0, -39.0, 1.0, 0.0]], s=w425, f=dbl[][] [[-8.43, -48.0, 4.0, 4.0], [-5.62, -45.0, 4.0, 4.0], [-2.81, -42.0, 4.0, 4.0], [0.0, -39.0, 1.0, 1.0], [-8.43, -62.0, 4.0, 0.0], [-5.62, -59.0, 4.0, 0.0], [-2.81, -56.0, 4.0, 0.0], [0.0, -53.0, 1.0, 0.0]]) -> (s? t:f=w422:dbl[][])
        n161 = Index Array(array=w459, index=2) -> (element=w455:dbl)
        n162 = call-dynamic "Z Go.vi"("error in (no error)"=w451, "Speed"=20.0, "Position"=0.0, "Motion in"=w448) -> ("error out"=w447:errorcluster, "Motion out"=w454:refnum<class "Motion.lvclass">)  [unwired: 6 in]
        n163 = call "Display Message to User2"("error in (no error)"=w447) -> ("error out"=w446:errorcluster)  [unwired: 9 in, 1 out]
        n164 = Add(x=w455, y=-2.5) -> (x+y=w456:dbl)
        n165 = call-dynamic "Z Go.vi"("error in (no error)"=w446, "Speed"=20.0, "Position"=w456, "Motion in"=w454) -> ("error out"=w444:errorcluster, "Motion out"=w445:refnum<class "Motion.lvclass">)  [unwired: 6 in]
        n166 = call-dynamic "Connect.vi"("Ultimus V in"=refnum<class "Ultimus V2.lvclass"> refnum ("Ultimus V2.lvclass")) -> ("Ultimus V out"=w442:refnum<class "Ultimus V2.lvclass">)  [unwired: 9 in, 1 out]
        n167 = case shown="True" w434 {
          tunnel: w445 -> [w485 w586]
          tunnel: w444 -> [w486 w585]
          tunnel: [w484 w584] -> w439
          tunnel: [w486 w583] -> w437
          tunnel: w433 -> [w481 w577]
          tunnel: w443 -> [w480 w582]
          tunnel: w442 -> [w482 w581]
          tunnel: [w483 w580] -> w440
          tunnel: w432 -> [w479 w579]
          tunnel: w422 -> [w478 _]
          tunnel: "Needle Height Compenstation\n(glue gap)" -> [w477 w578]
          tunnel: "check height?" -> [w476 w575]
          frame False {
            # "two sensor, Sensor B then A"
            n168 = for {
              N: w479 -> [_]
              tunnel: w485 -> [w502]
              tunnel: [w501] -> w483
              tunnel: [w500] -> w484
              tunnel: w482 -> [w499]
              tunnel: w481 -> [w498] mode=indexing
              tunnel: w480 -> [w492]
              tunnel: w478 -> [w494]
              tunnel: w477 -> [w488]
              tunnel: w476 -> [w487]
              i -> [w490]
              # "four\nloops"
              n169 = Multiply(x=4, y=w490) -> (x*y=w489:i32)
              n170 = Array Subset(array=w494, index (row)=w489, length (row)=4 ("length"), index (col)=0, length (col)=3 ("length")) -> (w493:dbl[][])
              "GlueBox" <- w493
              n171 = for {
                N: 4 -> [_]
                tunnel: w502 -> [w562]
                tunnel: [w553] -> w501
                tunnel: [w548] -> w500
                tunnel: w499 -> [w540]
                tunnel: w498 -> [w518]
                tunnel: w493 -> [w515] mode=indexing
                tunnel: w492 -> [w521]
                tunnel: w488 -> [w507]
                tunnel: w487 -> [w504]
                n172 = Index Array(array=w515, index=0) -> (element=w537:dbl)
                n173 = Index Array(array=w515, index=1) -> (element=w536:dbl)
                n174 = Array Subset(array=w518, index=0, length=2) -> (w520:dbl[])
                n175 = Add(x=w520, y=w521) -> (x+y=w519:dbl[])
                n176 = Absolute Value(x=w537) -> (abs(x)=w535:dbl)
                n177 = Absolute Value(x=w536) -> (abs(x)=w533:dbl)
                n178 = Add(x=w519, y=w515) -> (x+y=w530:dbl[])
                n179 = Multiply(x=w533, y=2.0) -> (x*y=w511:dbl)
                n180 = Multiply(x=w535, y=2.0) -> (x*y=w512:dbl)
                n181 = Multiply(x=w511, y=-1.0) -> (x*y=w523:dbl)
                n182 = Build Array(0.0 ("element"), w511) -> (w531:dbl[])
                n183 = Build Array(w512, 0.0 ("element")) -> (w528:dbl[])
                n184 = Build Array(0.0 ("element"), w523) -> (w509:dbl[])
                n185 = Add(x=w530, y=w531) -> (x+y=w527:dbl[])
                n186 = Add(x=w527, y=w528) -> (x+y=w510:dbl[])
                n187 = call-dynamic "XY Go.vi"("Speed"=200.0, "XY"=w530, "Motion in"=w562) -> ("error out"=w513:errorcluster, "Motion out"=w561:refnum<class "Motion.lvclass">)  [unwired: 7 in]
                n188 = Add(x=w510, y=w509) -> (x+y=w508:dbl[])
                n189 = Index Array(array=w518, index=2) -> (element=w517:dbl)
                n190 = Index Array(array=w515, index=2) -> (element=w514:dbl)
                n191 = Add(x=w517, y=w507) -> (x+y=w546:dbl)
                n192 = Build Array(w527, w510, w508, w530) -> (w522:dbl[][])
                "appended array" <- w522
                n193 = call-dynamic "Z Go.vi"("error in (no error)"=w513, "Speed"=5.0, "Position"=w546, "Motion in"=w561) -> ("error out"=w506:errorcluster, "Motion out"=w556:refnum<class "Motion.lvclass">)  [unwired: 6 in]
                n194 = case shown="True" w504 {
                  tunnel: w506 -> [w566 w568]
                  tunnel: [w566 w567] -> w505
                  frame False {
                  }
                  frame True {
                    n195 = call "Display Message to User11"("error in (no error)"=w568) -> ("error out"=w567:errorcluster)  [unwired: 9 in, 1 out]
                  }
                }
                n196 = call "vacuum.vi"("error in (no error)"=w505, "Vacuum Setting (0000)"=i64 100, "Ultimus V in"=w540) -> ("error out"=w559:errorcluster, "Ultimus V out"=w543:refnum<class "Ultimus V2.lvclass">)  [unwired: 7 in]
                n197 = call-dynamic "Pressure.vi"("error in (no error)"=w559, "Pressure"=i16 20, "Ultimus V in"=w543) -> ("error out"=w560:errorcluster, "Ultimus V out"=w542:refnum<class "Ultimus V2.lvclass">)  [unwired: 7 in]
                n198 = call-dynamic "Dispense.vi"("error in (no error)"=w560, "Ultimus V in"=w542) -> ("error out"=w555:errorcluster, "Ultimus V out"=w541:refnum<class "Ultimus V2.lvclass">)  [unwired: 8 in]
                n199 = for {
                  N: w514 -> [_]
                  tunnel: w556 -> [w574]
                  tunnel: w555 -> [w573]
                  tunnel: [w572] -> w554
                  tunnel: [w571] -> w552
                  tunnel: w522 -> [w570] mode=indexing
                  (unwired) 4.5 ("Speed")
                  n200 = call-dynamic "XY Go.vi"("error in (no error)"=w573, "Speed"=4.5, "XY"=w570, "Motion in"=w574) -> ("error out"=w572:errorcluster, "Motion out"=w571:refnum<class "Motion.lvclass">)  [unwired: 6 in]
                }
                n201 = Add(x=w546, y=-2.0) -> (x+y=w549:dbl)
                n202 = call-dynamic "Dispense.vi"("error in (no error)"=w554, "Ultimus V in"=w541) -> ("error out"=w547:errorcluster, "Ultimus V out"=w553:refnum<class "Ultimus V2.lvclass">)  [unwired: 8 in]
                n203 = call-dynamic "Z Go.vi"("error in (no error)"=w547, "Speed"=10.0, "Position"=w549, "Motion in"=w552) -> ("Motion out"=w548:refnum<class "Motion.lvclass">)  [unwired: 6 in, 1 out]
              }
            }
          }
          frame True {
            n204 = case shown="True" w575 {
              tunnel: w577 -> [w587 w591]
              tunnel: [w587 w588] -> w576
              frame False {
              }
              frame True {
                n205 = Array Subset(array=w591, index (row)=12 ("index"), length (row)=4 ("length")) -> (w588:dbl[][])  [unwired: 2 in]
              }
            }
            n206 = for {
              N: w579 -> [_]
              tunnel: w586 -> [w629]
              tunnel: w585 -> [w628]
              tunnel: [w613] -> w580
              tunnel: [w612] -> w584
              tunnel: [w611] -> w583
              tunnel: w576 -> [w599] mode=indexing
              tunnel: w582 -> [w598]
              tunnel: w581 -> [w597]
              tunnel: w578 -> [w595]
              tunnel: w575 -> [w592]
              # "move the glue in x-dir\n0.1 mm closer to center"
              n207 = Index Array(array=w599, index=2) -> (element=w600:dbl)
              n208 = Add(x=w599, y=w598) -> (x+y=w627:dbl[])
              n209 = Build Array(0.0 ("element"), 3.3 ("element")) -> (w632:dbl[])
              n210 = Subtract(x=w627, y=w632) -> (x-y=w633:dbl[])
              n211 = Add(x=w600, y=w595) -> (x+y=w601:dbl)
              n212 = Add(x=w627, y=w632) -> (x+y=w609:dbl[])
              n213 = call-dynamic "XY Go.vi"("error in (no error)"=w628, "Speed"=200.0, "XY"=w633, "Motion in"=w629) -> ("error out"=w614:errorcluster, "Motion out"=w607:refnum<class "Motion.lvclass">)  [unwired: 6 in]
              n214 = call-dynamic "Z Go.vi"("error in (no error)"=w614, "Speed"=5.0, "Position"=w601, "Motion in"=w607) -> ("error out"=w594:errorcluster)  [unwired: 6 in, 1 out]
              n215 = case shown="True" w592 {
                tunnel: w594 -> [w634 w636]
                tunnel: [w634 w635] -> w593
                frame False {
                }
                frame True {
                  n216 = call "Display Message to User7"("error in (no error)"=w636) -> ("error out"=w635:errorcluster)  [unwired: 9 in, 1 out]
                }
              }
              n217 = call "vacuum.vi"("error in (no error)"=w593, "Vacuum Setting (0000)"=i64 100, "Ultimus V in"=w597) -> ("error out"=w624:errorcluster, "Ultimus V out"=w619:refnum<class "Ultimus V2.lvclass">)  [unwired: 7 in]
              n218 = call-dynamic "Pressure.vi"("error in (no error)"=w624, "Pressure"=i16 20, "Ultimus V in"=w619) -> ("error out"=w625:errorcluster, "Ultimus V out"=w616:refnum<class "Ultimus V2.lvclass">)  [unwired: 7 in]
              n219 = call-dynamic "Dispense.vi"("error in (no error)"=w625, "Ultimus V in"=w616) -> ("error out"=w608:errorcluster, "Ultimus V out"=w615:refnum<class "Ultimus V2.lvclass">)  [unwired: 8 in]
              n220 = call "Time Delay"("error in (no error)"=w608) -> ("error out"=w606:errorcluster)  [unwired: 10 in]
              n221 = call-dynamic "XY Go.vi"("error in (no error)"=w606, "Speed"=5.0, "XY"=w609, "Motion in"=w607) -> ("error out"=w605:errorcluster, "Motion out"=w603:refnum<class "Motion.lvclass">)  [unwired: 6 in]
              n222 = call "Time Delay3"("error in (no error)"=w605) -> ("error out"=w604:errorcluster)  [unwired: 10 in]
              n223 = call "Time Delay2"("error in (no error)"=w606) -> ("error out"=w618:errorcluster)  [unwired: 10 in]
              n224 = call-dynamic "Dispense.vi"("error in (no error)"=w618, "Ultimus V in"=w615) -> ("Ultimus V out"=w613:refnum<class "Ultimus V2.lvclass">)  [unwired: 8 in, 1 out]
              n225 = Add(x=w601, y=-2.5) -> (x+y=w622:dbl)
              n226 = call-dynamic "Z Go.vi"("error in (no error)"=w604, "Speed"=10.0, "Position"=w622, "Motion in"=w603) -> ("error out"=w611:errorcluster, "Motion out"=w612:refnum<class "Motion.lvclass">)  [unwired: 6 in]
            }
          }
        }
        n227 = call-dynamic "Disconnect.vi"("Ultimus V in"=w440) -> ()  [unwired: 9 in, 1 out]
        n228 = call "XYZTheta Go.vi"("error in (no error)"=w437, "XYZTheta In"=dbl[] [800.0, 800.0, 0.0, 0.1], "Motion in"=w439) -> ("error out"=w438:errorcluster, "Motion out"=w435:refnum<class "Motion.lvclass">)  [unwired: 6 in, 1 out]
        n229 = call "Display Message to User3"("error in (no error)"=w438) -> ()  [unwired: 9 in, 2 out]
      }
      event "Needle Alignment": Value Change {
        (unwired) "Needle Alignment in progress ...." ("String")
        # "first needle park position\nneedle gap on Z value : 0.5 mm"
        # "Syringe-camera offset"
        n230 = event-data() -> ()  [unwired: 1 in, 6 out]
        n231 = call-poly <vilib>:"Read Delimited Spreadsheet.vi"("file path (dialog if empty)"=path "D:/INTT/V1/Assembly Data/Tool Offsets/Dispense Tip Offset.txt", "number of rows (all:-1)"=-1) -> ("first row"=w677:dbl[])  [unwired: 8 in, 5 out]
        n232 = Build Array(11.75, -25, 0.5 ("element"), 0.0 ("element")) -> (w670:dbl[])
        n233 = Index Array(array=w677, index #1=0 ("index"), index #2=1 ("index")) -> (element #1=w672:dbl, element #2=w669:dbl)
        n234 = Build Array(w672, w669, 0.0 ("element"), 0.0 ("element")) -> (w639:dbl[])
        n235 = Add(x=w639, y=w670) -> (x+y=w663:dbl[])
        n236 = Add(x=w662, y=w663) -> (x+y=w664:dbl[])
        n237 = call "XYZTheta Go.vi"("XYZTheta In"=w664, "Motion in"=w654) -> ("error out"=w668:errorcluster, "XYZTheta Out"=w644:dbl[], "Motion out"=w653:refnum<class "Motion.lvclass">)  [unwired: 7 in]
        n238 = call "Display Message to User10"("error in (no error)"=w668) -> ("error out"=w665:errorcluster)  [unwired: 9 in, 1 out]
        n239 = call-dynamic "Z Go.vi"("error in (no error)"=w665, "Speed"=20.0, "Position"=0.0, "Motion in"=w653) -> ("Motion out"=w652:refnum<class "Motion.lvclass">)  [unwired: 6 in, 1 out]
        n240 = Replace Array Subset(array=w644, new element=0.0 ("new element/subarray"), index=2) -> (w641:dbl[])
        n241 = call "Joystick and Camera - external Connection.vi"("Motion in"=w652, "XYZTheta"=w641, "Measurement Point"="Touch Needle on a surface") -> ("Motion out"=w650:refnum<class "Motion.lvclass">, "Gantry"=w640:dbl[])  [unwired: 4 in, 2 out]
        n242 = Subtract(x=w640, y=w639) -> (x-y=w638:dbl[])
        n243 = call "Joystick and Camera - external Connection.vi"("Motion in"=w650, "XYZTheta"=w638, "Measurement Point"="Measure the touch spot with camera") -> ("Motion out"=w646:refnum<class "Motion.lvclass">, "Gantry"=w649:dbl[])  [unwired: 4 in, 2 out]
        n244 = Subtract(x=w640, y=w649) -> (x-y=w648:dbl[])
        n245 = call-poly <vilib>:"Write Delimited Spreadsheet.vi"("file path (dialog if empty)"=path "D:/INTT/V1/Assembly Data/Tool Offsets/Dispense Tip Offset.txt", "1D data"=w648, "append to file? (new file:F)"=FALSE) -> ()  [unwired: 11 in, 2 out]
      }
      event "Pick and place": Value Change {
        (unwired) "PICK and PLACE samples ..." ("String")
        (unwired) -21.3804 ("new element/subarray")
        n246 = event-data() -> ()  [unwired: 1 in, 6 out]
        n247 = call-poly <vilib>:"Read Delimited Spreadsheet.vi"("file path (dialog if empty)"=path "D:/INTT/V1/Assembly Data/Tool Offsets/Bellows Tool Offset.txt", "number of rows (all:-1)"=-1) -> ("first row"=w706:dbl[])  [unwired: 8 in, 5 out]
        n248 = Select(t=1, s=w698, f=w694) -> (s? t:f=w711:i32)
        n249 = Index Array(array=w706, index #1=0 ("index"), index #2=1 ("index"), index #3=2 ("index")) -> (element #1=w702:dbl, element #2=w701:dbl, element #3=w700:dbl)
        n250 = case shown="True" w690 {
          tunnel: [w712 w715] -> w689
          tunnel: w685 -> [w712 w714]
          frame False {
          }
          frame True {
            # "sensor A"
            # "sensor B"
            n251 = Index Array(array=w714, index=0) -> (element=w713:i32)
            n252 = Index Array(array=w714, index=1) -> (element=w716:i32)
            n253 = Build Array(w716, w713) -> (w715:i32[])
          }
        }
        n254 = for {
          N: w711 -> [_]
          tunnel: w694 -> [w757]
          tunnel: w695 -> [w753]
          tunnel: w709 -> [w777]
          tunnel: [w765] -> w699
          tunnel: w696 -> [w775] mode=indexing
          tunnel: [w734] -> w688
          tunnel: w687 -> [w741]
          tunnel: w702 -> [w767]
          tunnel: w701 -> [w766]
          tunnel: w697 -> [w750]
          tunnel: w700 -> [w764]
          tunnel: w698 -> [w726]
          tunnel: w689 -> [w743]
          tunnel: "VacChannel for sample" -> [w729]
          tunnel: "check height? 2" -> [w720]
          tunnel: "check height? 2" -> [w719]
          i -> [w742]
          w728 = 0
          # "if chips, do one pickup tool and multiple samples;\nif sensors, one pickup tool for one sample ( so 2->2);"
          # "build a fake 2d arrays"
          # "sensor"
          # "chip pickup tool"
          # "pickup tool height offset"
          # "Pick up PICKUP TOOL"
          # "Pick up CHIPs/Sensor and place on HDI"
          n255 = Select(t=w757, s=w726, f=1) -> (s? t:f=w756:i32)
          n256 = Build Array(w767, w766, w764, 0.0 ("element")) -> (w762:dbl[])
          n257 = Add(x=w775, y=w762) -> (x+y=w763:dbl[])
          n258 = call "XYZTheta-2Zspeed Go.vi"("XYZTheta In"=w763, "Motion in"=w777) -> ("error out"=w740:errorcluster, "Motion out"=w776:refnum<class "Motion.lvclass">)  [unwired: 7 in, 1 out]
          n259 = Select(t=-18.52 ("new element/subarray"), s=w726, f=-13.13 ("t")) -> (s? t:f=w758:dbl)
          n260 = call-dynamic "Digital Write 1 Channel.vi"("DAQ Module"=w728, "error constant"=w740, "Value"=TRUE, "Channel"=0, "NI-DAQ.lvclass"=w741) -> ("error IO"=w725:errorcluster, "NI-DAQ.lvclass 2"=w739:refnum<class "NI-DAQ.lvclass">)  [unwired: 5 in]
          n261 = Replace Array Subset(array=w762, new element=w758, index=2) -> (w760:dbl[])
          n262 = Index Array(array=w753, index (row)=w742) -> (element=w752:dbl[])  [unwired: 1 in]
          n263 = Index Array(array=w743, index=w742) -> (element=w736:i32)
          n264 = call "Time Delay8"("error in (no error)"=w725) -> ("error out"=w773:errorcluster)  [unwired: 10 in]
          n265 = Build Array(w752, w752) -> (w751:dbl[][])
          n266 = Select(t=w753, s=w726, f=w751) -> (s? t:f=w754:dbl[][])
          n267 = Index Array(array=w750, index (row)=w742) -> (element=w749:dbl[])  [unwired: 1 in]
          n268 = Build Array(w749, w749) -> (w748:dbl[][])
          n269 = Select(t=w750, s=w726, f=w748) -> (s? t:f=w722:dbl[][])
          n270 = case shown="False" w719 {
            tunnel: [w778 w780] -> w721
            tunnel: w722 -> [w778 w779]
            frame False {
            }
            frame True {
              n271 = Array Subset(array=w779, index (row)=12 ("index"), length (row)=4 ("length")) -> (w780:dbl[][])  [unwired: 2 in]
            }
          }
          n272 = Select(t="chip placement height compensation", s=w726, f=0.0) -> (s? t:f=w723:dbl)
          n273 = for {
            N: w756 -> [_]
            tunnel: w754 -> [w798] mode=indexing
            tunnel: w776 -> [w800]
            tunnel: w760 -> [w799]
            tunnel: w773 -> [w797]
            tunnel: [w796] -> w768
            tunnel: w728 -> [w795]
            tunnel: w739 -> [w794]
            tunnel: w721 -> [w791] mode=indexing
            tunnel: [w790] -> w759
            tunnel: w723 -> [w789]
            tunnel: w736 -> [w787]
            tunnel: w729 -> [w786]
            tunnel: [w785] -> w727
            tunnel: w726 -> [w784]
            tunnel: w720 -> [w783]
            n274 = flat-sequence {
              tunnel: w798 -> [w819]
              tunnel: [w821] -> w801
              tunnel: w800 -> [w820]
              tunnel: w799 -> [w818]
              tunnel: w797 -> [w816]
              tunnel: w795 -> [w809]
              tunnel: w794 -> [w813]
              tunnel: [w815] -> w793
              tunnel: [w807] -> w792
              tunnel: [w809] -> w788
              tunnel: w787 -> [w803]
              tunnel: w786 -> [w802]
              tunnel: w801 -> [w844]
              tunnel: [w843] -> w796
              tunnel: w799 -> [w841]
              tunnel: w793 -> [w842]
              tunnel: w792 -> [w827]
              tunnel: w791 -> [w840]
              tunnel: [w823] -> w790
              tunnel: w789 -> [w833]
              tunnel: w788 -> [w830]
              tunnel: w786 -> [w825]
              tunnel: [w824] -> w785
              tunnel: w784 -> [_]
              tunnel: w783 -> [w822]
              frame #0 {
                # "pickup sample from tray"
                n275 = Add(x=w819, y=w818) -> (x+y=w817:dbl[])
                n276 = call "XYZTheta-2Zspeed Go.vi"("error in (no error)"=w816, "XYZTheta In"=w817, "Motion in"=w820) -> ("error out"=w814:errorcluster, "Motion out"=w821:refnum<class "Motion.lvclass">)  [unwired: 6 in, 1 out]
                n277 = call "Time Delay4"("error in (no error)"=w814) -> ("error out"=w812:errorcluster)  [unwired: 10 in]
                n278 = call-dynamic "Digital Write 1 Channel.vi"("DAQ Module"=w809, "error constant"=w812, "Value"=FALSE, "Channel"=w803, "NI-DAQ.lvclass"=w813) -> ("error IO"=w811:errorcluster, "NI-DAQ.lvclass 2"=w808:refnum<class "NI-DAQ.lvclass">)  [unwired: 5 in]
                n279 = call "Time Delay11"("error in (no error)"=w811) -> ("error out"=w805:errorcluster)  [unwired: 10 in]
                n280 = call-dynamic "Digital Write 1 Channel.vi"("DAQ Module"=w809, "error constant"=w805, "Value"=TRUE, "Channel"=w802, "NI-DAQ.lvclass"=w808) -> ("error IO"=w804:errorcluster, "NI-DAQ.lvclass 2"=w807:refnum<class "NI-DAQ.lvclass">)  [unwired: 5 in]
                n281 = call "Time Delay5"("error in (no error)"=w804) -> ("error out"=w815:errorcluster)  [unwired: 10 in]
              }
              frame #1 {
                # "lift for chip/sensor thickness"
                # "place sample on HDI"
                n282 = Add(x=w840, y=w841) -> (x+y=w836:dbl[])
                n283 = Build Array(0.0 ("element"), 0.0 ("element"), w833, 0.0 ("element")) -> (w835:dbl[])
                n284 = Add(x=w836, y=w835) -> (x+y=w834:dbl[])
                n285 = call "XYZTheta-2Zspeed Go.vi"("error in (no error)"=w842, "XYZTheta In"=w834, "Motion in"=w844) -> ("error out"=w832:errorcluster, "Motion out"=w843:refnum<class "Motion.lvclass">)  [unwired: 6 in, 1 out]
                n286 = case shown="True" w822 {
                  tunnel: w832 -> [w845 w847]
                  tunnel: [w845 w846] -> w831
                  frame False {
                  }
                  frame True {
                    n287 = call "Display Message to User6"("error in (no error)"=w847) -> ("error out"=w846:errorcluster)  [unwired: 9 in, 1 out]
                  }
                }
                n288 = call "Time Delay6"("error in (no error)"=w831) -> ("error out"=w828:errorcluster)  [unwired: 10 in]
                n289 = call-dynamic "Digital Write 1 Channel.vi"("DAQ Module"=w830, "error constant"=w828, "Value"=FALSE, "Channel"=w825, "NI-DAQ.lvclass"=w827) -> ("error IO"=w829:errorcluster, "NI-DAQ.lvclass 2"=w824:refnum<class "NI-DAQ.lvclass">)  [unwired: 5 in]
                n290 = call "Time Delay7"("error in (no error)"=w829) -> ("error out"=w823:errorcluster)  [unwired: 10 in]
              }
            }
          }
          n291 = call "XYZTheta-2Zspeed Go.vi"("error in (no error)"=w759, "XYZTheta In"=w763, "Motion in"=w768) -> ("error out"=w724:errorcluster, "Motion out"=w772:refnum<class "Motion.lvclass">)  [unwired: 6 in, 1 out]
          n292 = call "Time Delay9"("error in (no error)"=w724) -> ("error out"=w732:errorcluster)  [unwired: 10 in]
          n293 = call-dynamic "Digital Write 1 Channel.vi"("DAQ Module"=0, "error constant"=w732, "Value"=FALSE, "Channel"=0, "NI-DAQ.lvclass"=w727) -> ("error IO"=w735:errorcluster, "NI-DAQ.lvclass 2"=w734:refnum<class "NI-DAQ.lvclass">)  [unwired: 5 in]
          n294 = call "Time Delay10"("error in (no error)"=w735) -> ("error out"=w769:errorcluster)  [unwired: 10 in]
          n295 = call-dynamic "Z Go.vi"("error in (no error)"=w769, "Speed"=10.0, "Position"=0.0 ("new element/subarray"), "Motion in"=w772) -> ("Motion out"=w765:refnum<class "Motion.lvclass">)  [unwired: 6 in, 1 out]
        }
      }
      event "GOTO": Value Change {
        (unwired) "GOING to a position" ("String")
        n296 = event-data() -> ()  [unwired: 1 in, 6 out]
        n297 = call "XYZTheta-2Zspeed Go.vi"("XYZTheta In"="Parking position", "Motion in"=w850) -> ("Motion out"=w849:refnum<class "Motion.lvclass">)  [unwired: 7 in, 2 out]
      }
      event "READ Position": Value Change {
        n298 = event-data() -> ()  [unwired: 1 in, 6 out]
        n299 = call-dynamic "Get Current Position.vi"("Motion in"=w871) -> ("XYZTheta Out"=→"Gantry current position":dbl[], "Motion out"=w870:refnum<class "Motion.lvclass">)  [unwired: 8 in, 1 out]
      }
      event "TrayVaccum": Value Change {
        n300 = event-data() -> ()  [unwired: 1 in, 6 out]
        n301 = call-dynamic "Digital Write Multiple Channels.vi"("DAQ Module"=0, "Values"="Values", "Indices"=w872, "NI-DAQ in"=w876) -> ("NI-DAQ out"=w875:refnum<class "NI-DAQ.lvclass">)  [unwired: 6 in, 1 out]
      }
    }
    "Measure HDI top-left" <- w34
    "Array" <- w14
    "Measured PickupTool position" <- w8
    n302 = feedback-in #1(w32) -> ()
    n303 = feedback-in #2(w34) -> ()
    n304 = feedback-in #3(w29) -> ()
    n305 = feedback-in #4(w22) -> ()
    n306 = feedback-in #5(w19) -> ()
    n307 = feedback-in #6(w8) -> ()
    n308 = feedback-in #7(w14) -> ()
    n309 = feedback-in #8(w27) -> ()
    "# of tasks excuted" <- w24
  }
  n310 = call-dynamic "Disconnect.vi"("I-O in"=w1) -> ()  [unwired: 9 in, 1 out]
  n311 = call-dynamic "Disconnect.vi"("Controller in"=w4) -> ()  [unwired: 9 in, 1 out]
